vi "Lockin-4461 -Patrick -State Arrayvi.vi"(10 "IV Curve Mode":bool, 11 "Channels: AO":T6={"AO amp (V)"=[0.0, 0.0, 0.0, 0.0, 0.0, 0.0, 0.0, 0.0], "AO DC (V)"=[0.0, 0.0, 0.0, 0.0, 0.0, 0.0, 0.0, 0.0], "AO f (Hz)"=[13.0, 13.0, 13.0, 13.0, 13.0, 13.0, 13.0, 13.0], "AO phi (deg)"=[0.0, 0.0, 0.0, 0.0, 0.0, 0.0, 0.0, 0.0], "function"=[enum."Sine Wave", enum."Sine Wave", enum."Sine Wave", enum."Sine Wave", enum."Sine Wave", enum."Sine Wave", enum."Sine Wave", enum."Sine Wave"]} {"AO f (Hz)" min=0.001 max=10000.0; "AO DC (V)" format="%#_6p"; "AO amp (V)" format="%#_6p"}) -> ()   [LabVIEW 2016]
uses:
  <vilib>/Analysis/4window.llb/windowTd.ctl
  <vilib>/measure/maspectr.llb/Power Spectrum and PSD Export Mode.ctl
  <vilib>/Utility/error.llb/DialogType.ctl
  <vilib>/Analysis/baseanly.llb/Mean (DBL).vi
  <vilib>/Analysis/2dsp.llb/Decimate (single shot).vi
  <vilib>/Analysis/2dsp.llb/Decimate (single shot, DBL).vi
  <userlib>/_OpenG.lib/array/array.llb/Empty 1D Array (Variant)__ogtk.vi
  <vilib>/Platform/browser.llb/Open URL in Default Browser (string).vi
  <userlib>/_OpenG.lib/error/error.llb/Filter Error Codes (Array)__ogtk.vi
  <userlib>/_OpenG.lib/array/array.llb/Empty 1D Array (DBL)__ogtk.vi
  <vilib>/measure/maspectr.llb/FFT Power Spectrum and PSD for N Chan.vi
  <vilib>/Waveform/WDTOps.llb/WDT Waveform to XY Pairs DBL.vi
  <vilib>/measure/NI_MAPro.lvlib
  <vilib>/Analysis/NI_AALBase.lvlib
  <vilib>/Utility/config.llb/NI_LVConfig.lvlib
  <vilib>/Analysis/NI_AALPro.lvlib
panel:
  in  "Tab Control 3":enum32{"Page 1"}(tab)
  in  "Bug":bool
  in  "Trigger":bool
  in  "Notes":string
  in  "Path":path=path "C:/Data/lockin"
  in  "EXIT":bool
  in  "RESET":bool
  in  "Save Data":bool
  out "X or R":dbl=6.757945856560922e-07 caption="X or R: Current (A) or Voltage (V)" format="%#.3p"
  out "Y or Theta":dbl=134.81038545044584 caption="Y or Theta: Current (A) or Voltage (V)" format="%.3p"
  in  "Display":enum16{"X and Y", "R and Theta"}(ring)=enum."R and Theta"
  in  "Channel":dbl min=0.0 max=7.0 step=1.0
  in  "Remote Mode":bool
  out "time and date":string="22:38:56.0   2016-12-22"
  out "DAQ mode string":string="USB 4431"
  out "time since trigger":dbl
  in  "mean":dbl[](array[numeric])=[2.3266197706225262]
  in  "Tab Control 2":T1(tab)
  in  "Output signals?":bool
  out "Signals Graph":waveform(dbl)[](graph)=[{"t0"=timestamp(3565309135.890656 s since 1904-01-01), "dt"=1.0, "Y"=array[7876 elements], "attributes"=variant("NI_ChannelName"=variant(string "Dev1/ai0"), "NI_UnitDescription"=variant(string "Volts"))}]
  out "Reference Graph":waveform(dbl)[](graph)=[{"t0"=timestamp(3565309136.0036526 s since 1904-01-01), "dt"=1.0, "Y"=array[7876 elements]}, {"t0"=timestamp(3565309136.0036526 s since 1904-01-01), "dt"=1.0, "Y"=array[7876 elements]}]
  in  "decimate graph":i32=1
  in  "Display n?":bool=TRUE
  out "Display X (or R)":waveform(dbl)[](graph)=[{"t0"=timestamp(3565309135.890656 s since 1904-01-01), "dt"=1.0, "Y"=[6.757945856560922e-07]}]
  out "Display Y (or Theta)":waveform(dbl)[](graph)=[{"t0"=timestamp(3565309135.890656 s since 1904-01-01), "dt"=1.0, "Y"=[134.81038545044584]}]
  out "XY Graph":cluster{dbl[], dbl[]}[](graph)=[{[0.0, -4.762748948158435e-07], [0.0, 4.794377400353947e-07]}]
  out "Results\n(X, Y, R, Theta, mean)":dbl[][](array[numeric])=[[-4.762748948158435e-07, 4.794377400353947e-07, 6.757945856560922e-07, 134.81038545044584, 2.3266197706225262]] format="%#_3p"
  out "PS Chart":dbl[][](graph)=[[-1411.497616925462, -1404.3790029743438, -1413.0961920610762, -1418.6418791322994, -1413.136726104145, -1413.4151534226191, -1417.9246313001065, -1424.6072395567076]]
  out "PS dB":cluster{"f0":dbl, "df":dbl, "magnitude":dbl[]}[](graph)
  in  "window":T2=1 items=["Rectangle"=0, "Hanning"=1, "Hamming"=2, "Blackman-Harris"=3, "Exact Blackman"=4, "Blackman"=5, "Flat Top"=6, "4 Term B-Harris "=7, "7 Term B-Harris"=8, "Low Sidelobe"=9, "Blackman Nuttall"=11, "Triangle"=30, "Bartlett-Hanning"=31, "Bohman"=32, "Parzen"=33, "Welch"=34, "Kaiser"=60, "Dolph-Chebyshev"=61, "Gaussian"=62]
  in  "averaging parameters":T3={"averaging mode"=enum."RMS averaging", "weighting mode"=enum."Exponential", "number of averages"=10} {"number of averages" min=1}
  in  "restart averaging (F)":bool
  in  "export mode":T4 items=["Power Spectrum", "Power Spectral Density"]
  in  "window parameter":dbl=nan
  out "averages\ncompleted":dbl=8319.0
  out "averaging done":bool=TRUE
  in  "Tab Control":T5(tab)=enum."DAQ Settings"
  in  "...............reset REF":bool
  in  "............zero offset":bool
  in  "....measure offset":bool
  in  "............all  f same":bool
  in  "..........reset signal":bool
  in  "60 Hz prefilter":bool
  in  "LP prefilter":bool
  in  "LP cutoff (Hz)":dbl=30.0
  in  "Channels: Lockin":T7={"REF f (Hz)"=[13.0], "REF phi (deg)"=[0.0]} {"REF phi (deg)" format="%#_3g"}
  in  "D":dbl=0.019999999999999997 format="%.2f"
  in  "I":dbl=0.6 format="%.2f"
  in  "P":dbl=0.5 format="%.2f"
  in  "autophase?\n(experimental)":bool
  out "filter fC (Hz)":dbl=0.5305164769729844
  in  "TC (s)":dbl=0.3 format="%#_6p"
  in  "order":i32=2
  in  "save config":bool
  in  "load config":bool
  in  "Instrument":u16(ring) items=["SIMULATE", "CF900", "DR200", "MNK", "PPMS1", "PPMS2", "THz1", "THz2"]
  in  "AO Configuration":T8(array[cluster])=[{"Output physical channels"="Dev1/ao0", "AO. Max"=3.5, "AO.Min"=-3.5}]
  in  "AI Configuration":T9(array[cluster])=[{"AI.Coupling"=enum."DC", "AI.Max"=10.0, "AI.Min"=-10.0, "Input physical channels"="Dev1/ai0"}, {"AI.Coupling"=enum."DC", "AI.Max"=10.0, "AI.Min"=-10.0, "Input physical channels"="Dev1/ai1"}]
  in  "#s":i32=7876
  in  "Fs":i32=102388
  in  "auto size":bool=TRUE
  in  "decimating factor":i32=1
  in  "AI Buffer Size (S)":i32=100
  out "dt":dbl=9.766769543305856e-06 format="%#_6p"
  in  "frequency multiplier":dbl=10000.0 format="%#_13g"
  out "sampling info":cluster{"Fs":i32, "#s":i32}={"Fs"=102388, "#s"=7876}
  in  "DAQ Type":enum16{"None", "USB 4431", "PXI 446x"}(ring)=enum."USB 4431"
  in  "Amplifiers":enum16{"None", "Krohn Hite", "Femto"}(ring)
  out "Current State":string="Exit"
  out "State History":string="Macro: Initialize\rData: Initialize\rInitialize Core Data\rUI: Initialize\rUI: Front Panel State\r4461: SETUP\r4461: CREATE TASKS\rError Handler\rMacro: Exit\rData: Cleanup\rExit"
  in  "offsets":dbl[](array[numeric])=[-2.856912612915039e-05, 0.0001668522834777832, 0.00010829269886016845, 0.0027965894103050234, 0.002931471037864685, 0.0029329052329063418] format="%#.2p"
  in  "Gain":dbl[](array[numeric])=[1.0, 1.0, 1.0, 1.0, 1.0, 1.0, 1.0, 1.0]
  out "phase log":dbl[](array[numeric]) format="%.1f"
  out "AI tasks":i32
  out "AO tasks":i32
  out "error":errorcluster={"status"=TRUE, "code"=-89131, "source"="DAQmx Start Task.vi:7220017<append>\n<B>Property: </B>Start.DigEdge.Src\n<B>Property: </B>Start.DigEdge.Edge\n<B>Source Device: </B>Dev1\n<B>Source Terminal: </B>ai/StartTrigger\n\n<B>Task Name: </B>_unnamedTask<2B>"}
  # "´"
  # "Multichannel Lockin v2016/12/15 v2.0"
  # "plot 0    = AI0 f0\nplot 1    = Ai1 f0\n...\nplot N-1  = AIN f0\n\nplot N    = AI0 f1\nplot N+1  = AI1 f1\n..."
  # "AO Settings"
  # "Lockin Settings"
  # "prefilters"
  # "lockin filter"
  # "autophase"
  # "0"
  # "1"
  # "2"
  # "3"
  # "4"
  # "5"
  # "6"
  # "7"
  # "configuration"
  # "sampling"
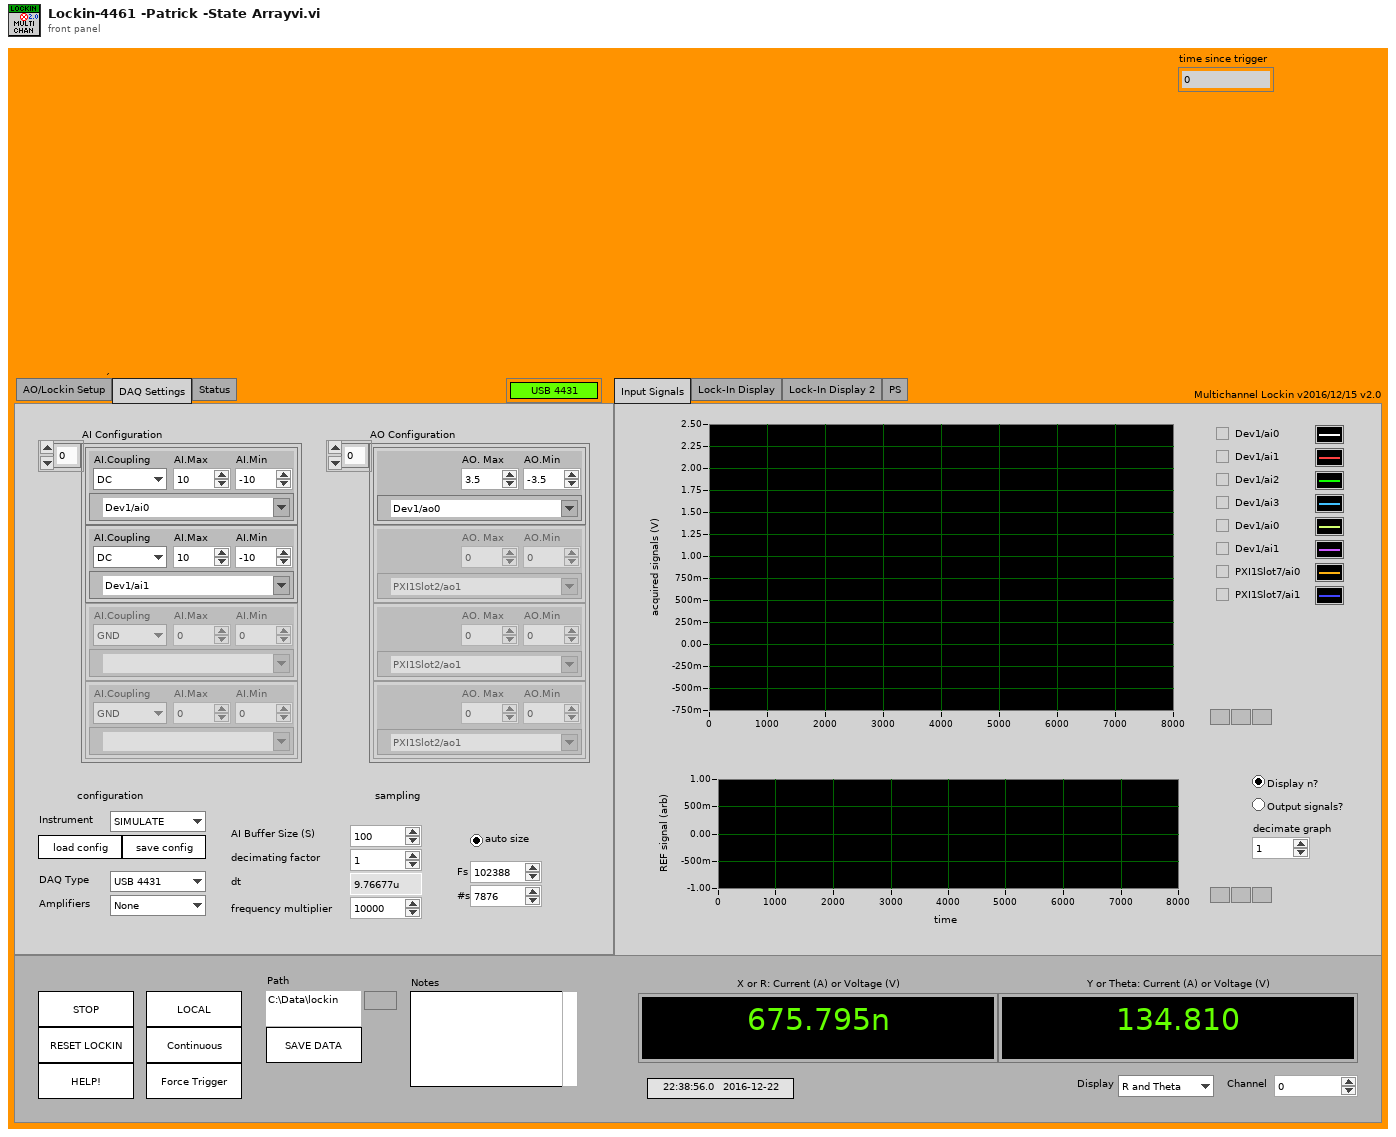
[diagram p1: front panel]
types:
  T1 = enum32{"Input Signals", "Lock-In Display", "Lock-In Display 2", "PS"}
  T2 = typedef "NI_AALPro.lvlib/windowTd.ctl" = u32
  T3 = cluster{"averaging mode":enum16{"No averaging", "Vector averaging", "RMS averaging", "Peak hold"}, "weighting mode":enum16{"Linear", "Exponential"}, "number of averages":u32}
  T4 = typedef "NI_MAPro.lvlib/Power Spectrum and PSD Export Mode.ctl" = u16
  T5 = enum32{"AO/Lockin Setup", "DAQ Settings", "Status"}
  T6 = cluster{"AO amp (V)":dbl[], "AO DC (V)":dbl[], "AO f (Hz)":dbl[], "AO phi (deg)":dbl[], "function":enum16{"Sine Wave", "Triangle Wave", "Square Wave", "Sawtooth Wave"}[]}
  T7 = cluster{"REF f (Hz)":dbl[], "REF phi (deg)":dbl[]}
  T8 = cluster{"Output physical channels":tag, "AO. Max":dbl, "AO.Min":dbl}[]
  T9 = cluster{"AI.Coupling":enum16{"AC", "DC", "GND"}, "AI.Max":dbl, "AI.Min":dbl, "Input physical channels":tag}[]
  T10 = enum32{"invalid app kind", "Development System", "Run Time System", "Student Edition", "Embedded LabVIEW", "Evaluation", "Custom"}
  T11 = enum32{"Invalid", "Standard", "Closed", "Hidden", "Minimized", "Maximized"}
  T12 = enum32{"Input Signals", "Lock-In Display", "Lock-In Display 2", "PS", "FFT"}
  T13 = cluster{"Core":cluster{"Current VI Reference":refnum<vi>, "Close Panel on Exit?":bool}, "Error":bool, "Your string data":string, "AI task":refnum<k21>[], "AO task":refnum<k21>[], "Input Signals":waveform(dbl)[], "Ouput Signals":waveform(dbl)[], "REF":waveform(dbl)[], "sampling info":cluster{"Fs":dbl, "#s":dbl}, "Tasks":string[]}
  T14 = typedef "DialogType.ctl" = u16
  T15 = cluster{"Current VI Reference":refnum<vi>, "Close Panel on Exit?":bool}
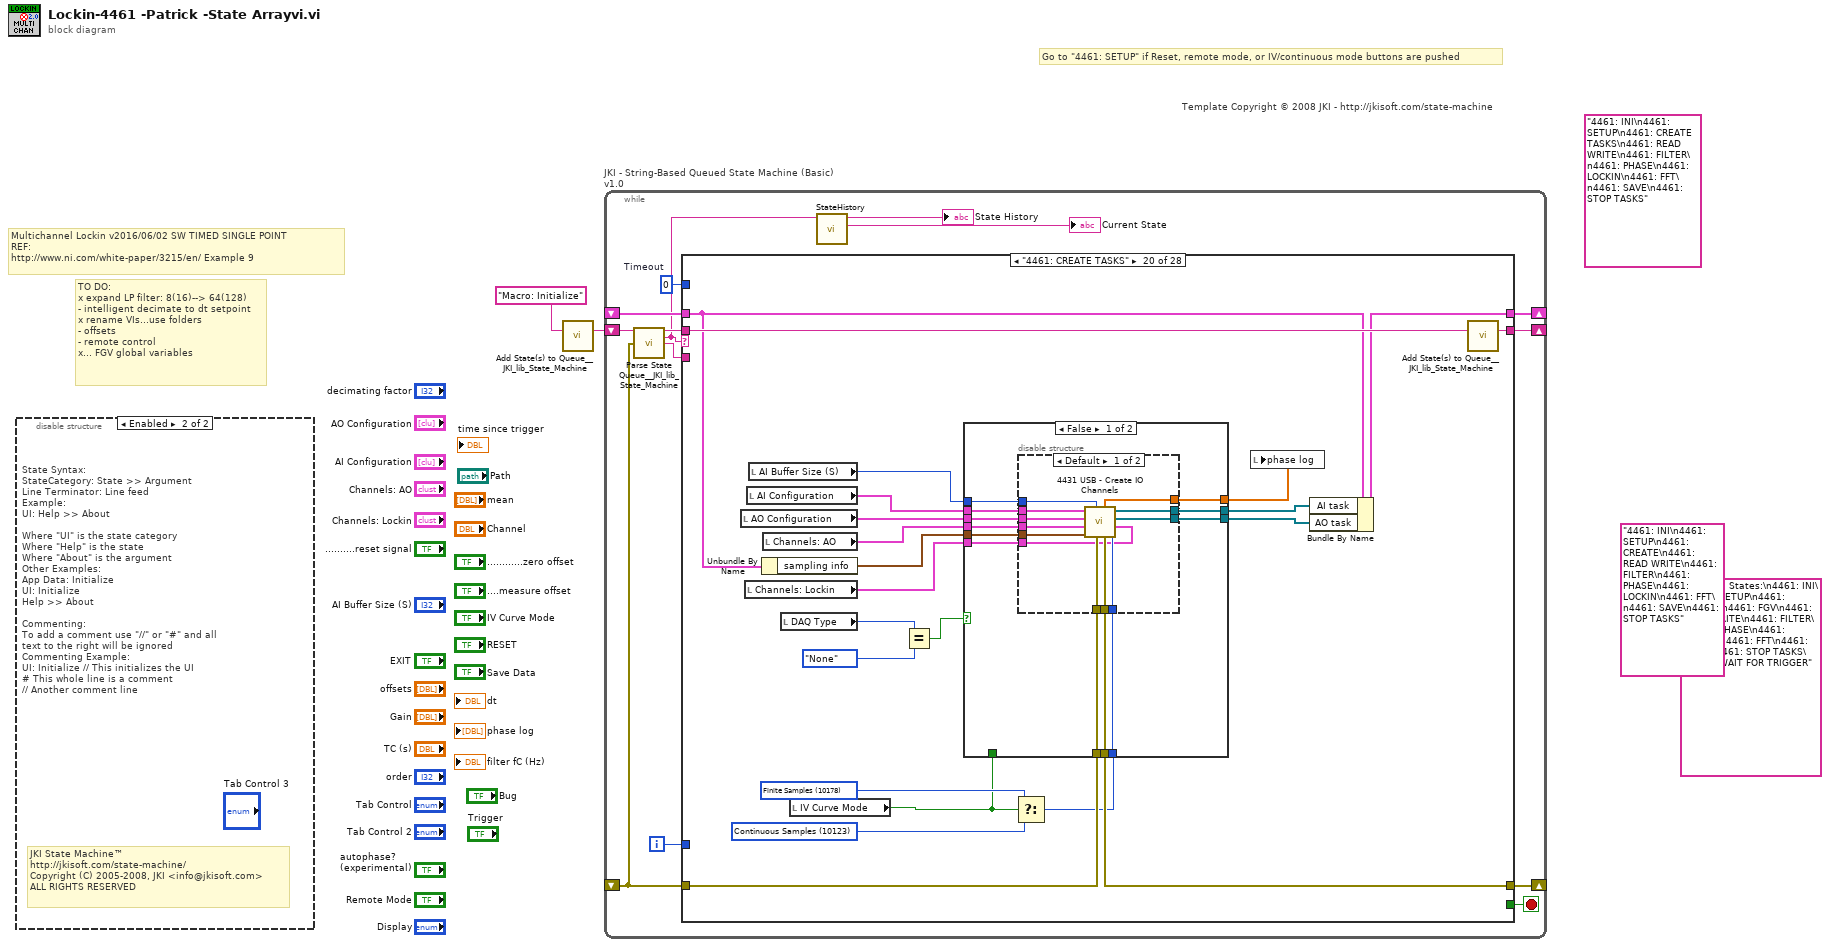
[diagram p0: block diagram]
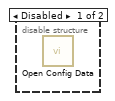
[diagram p2: hidden frame]
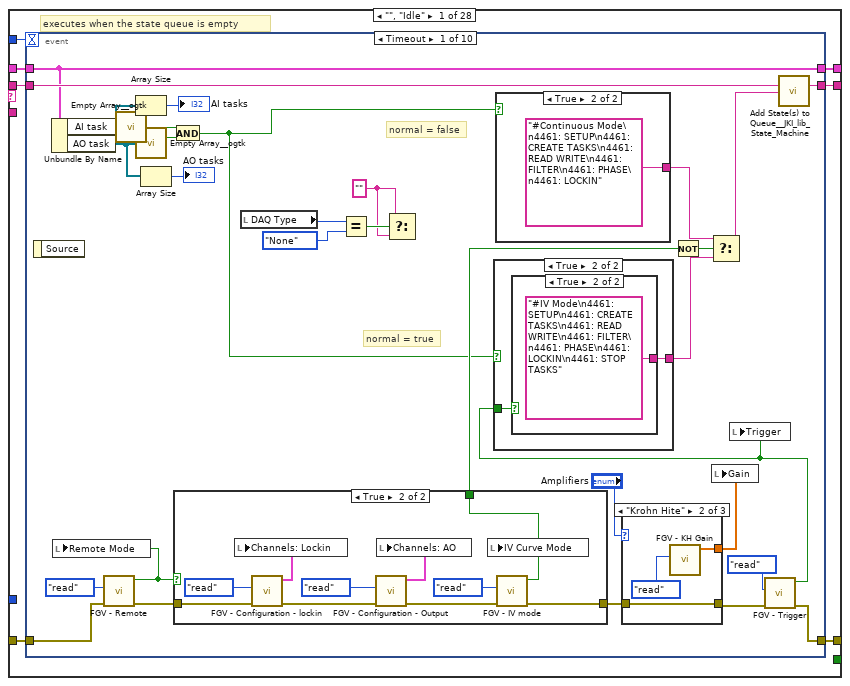
[diagram p3: hidden frame]
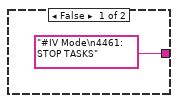
[diagram p4: hidden frame]
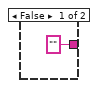
[diagram p5: hidden frame]
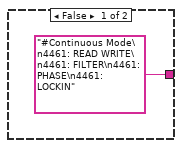
[diagram p6: hidden frame]
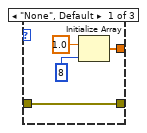
[diagram p7: hidden frame]
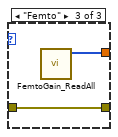
[diagram p8: hidden frame]
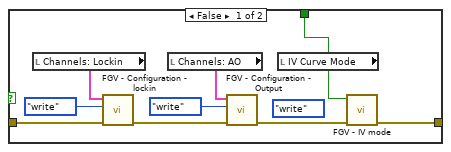
[diagram p9: hidden frame]
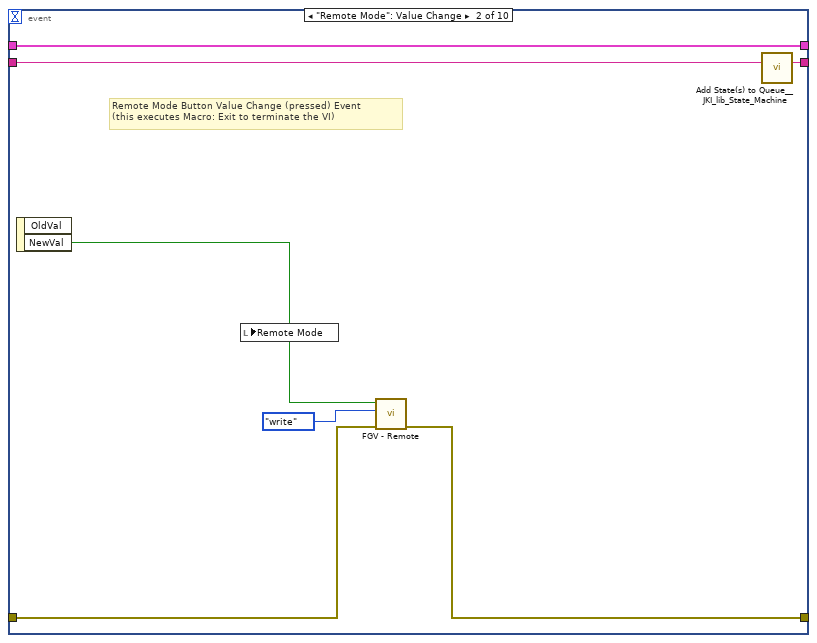
[diagram p10: hidden frame]
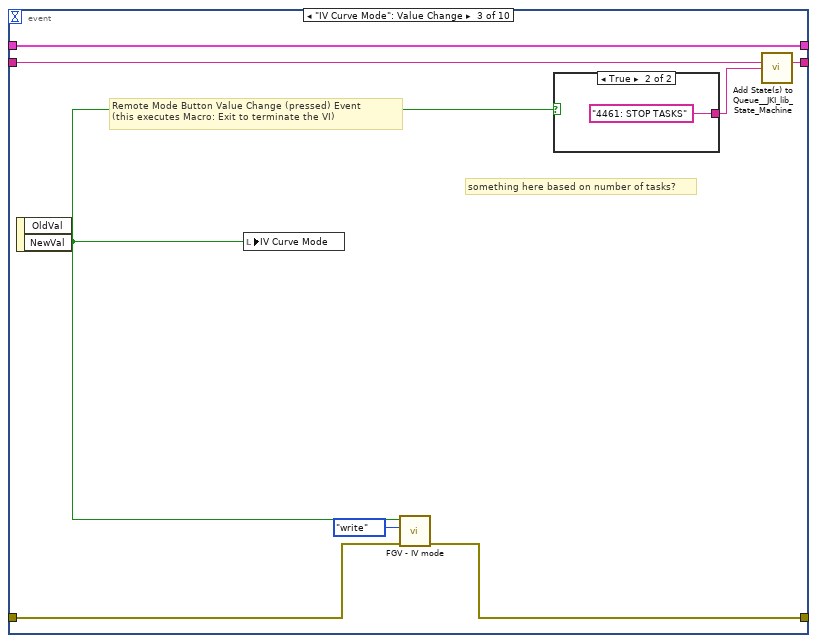
[diagram p11: hidden frame]
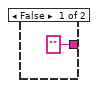
[diagram p12: hidden frame]
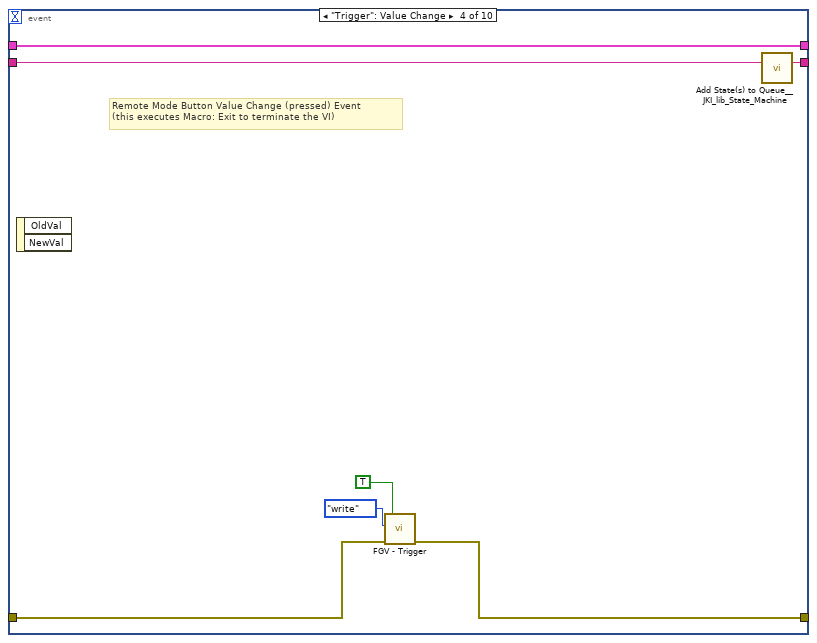
[diagram p13: hidden frame]
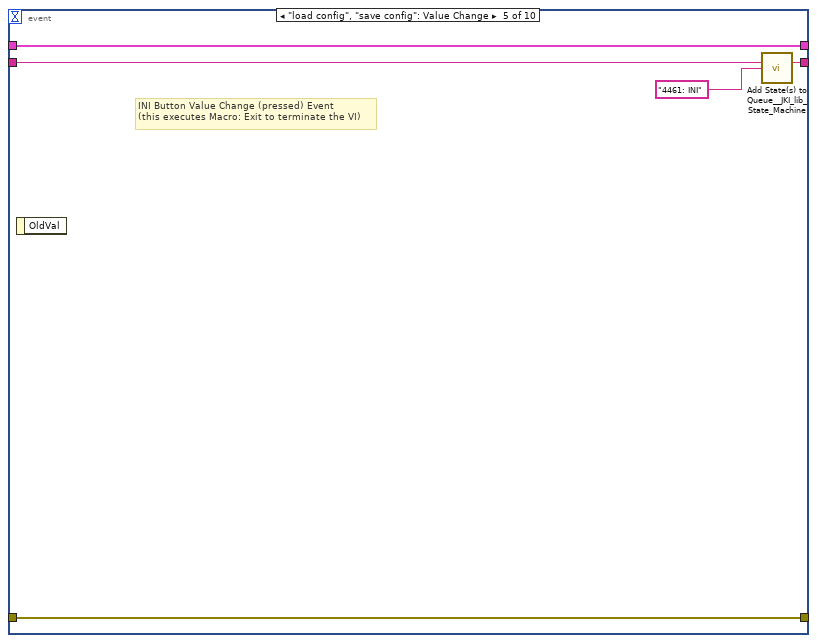
[diagram p14: hidden frame]
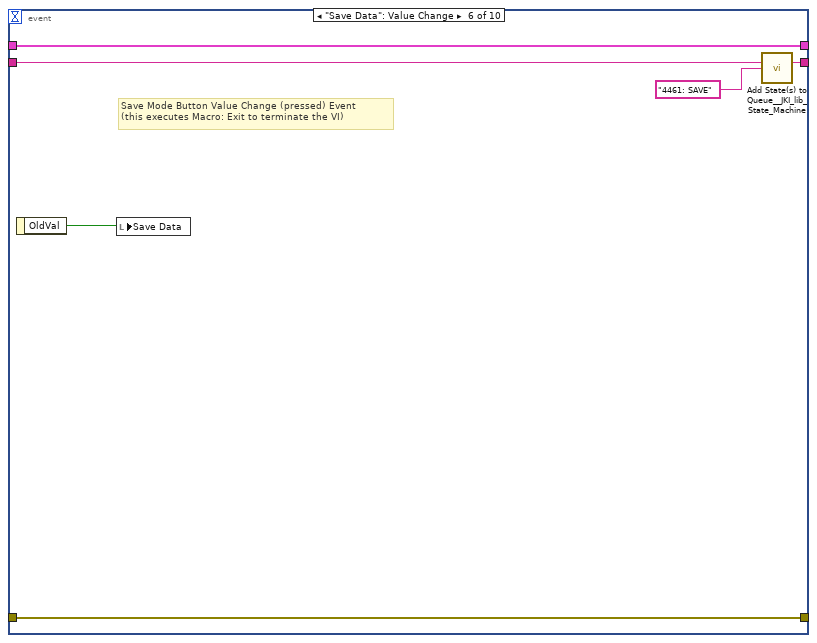
[diagram p15: hidden frame]
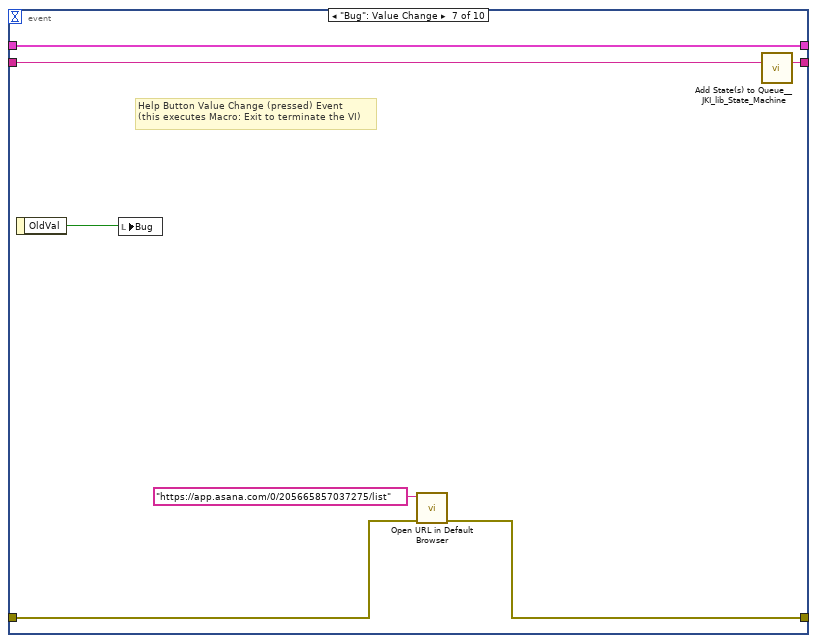
[diagram p16: hidden frame]
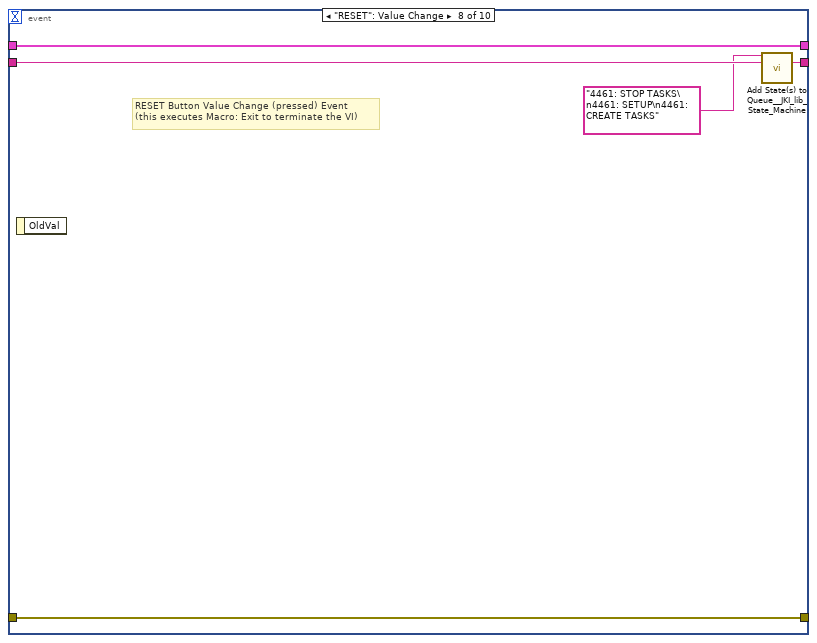
[diagram p17: hidden frame]
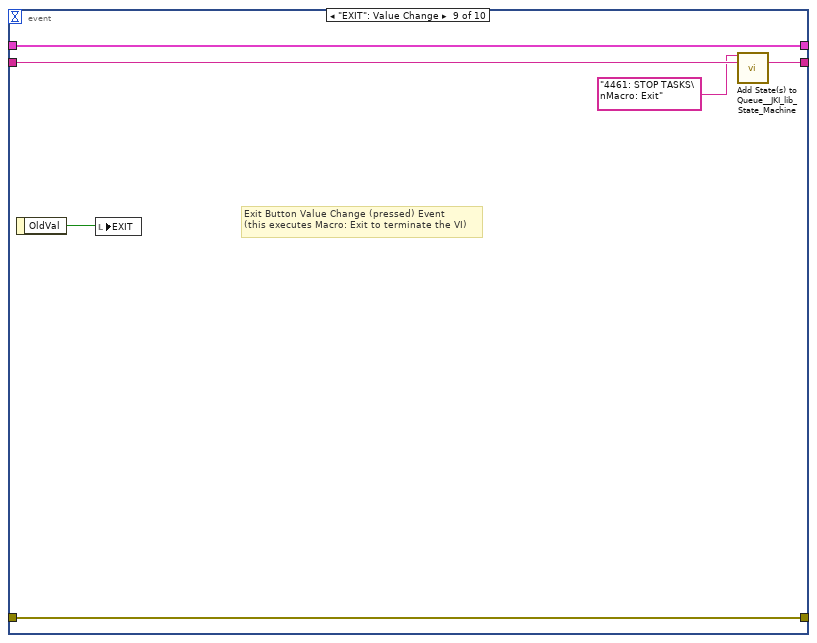
[diagram p18: hidden frame]
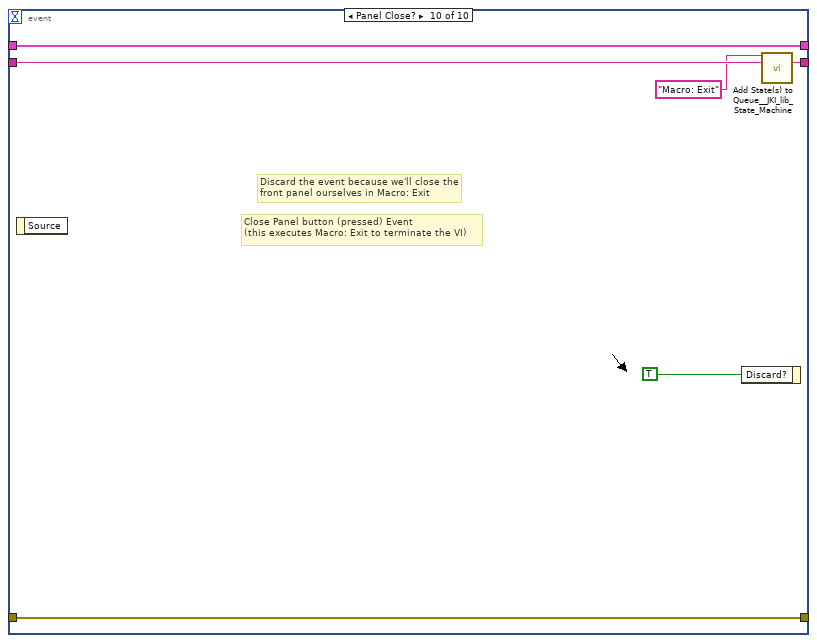
[diagram p19: hidden frame]
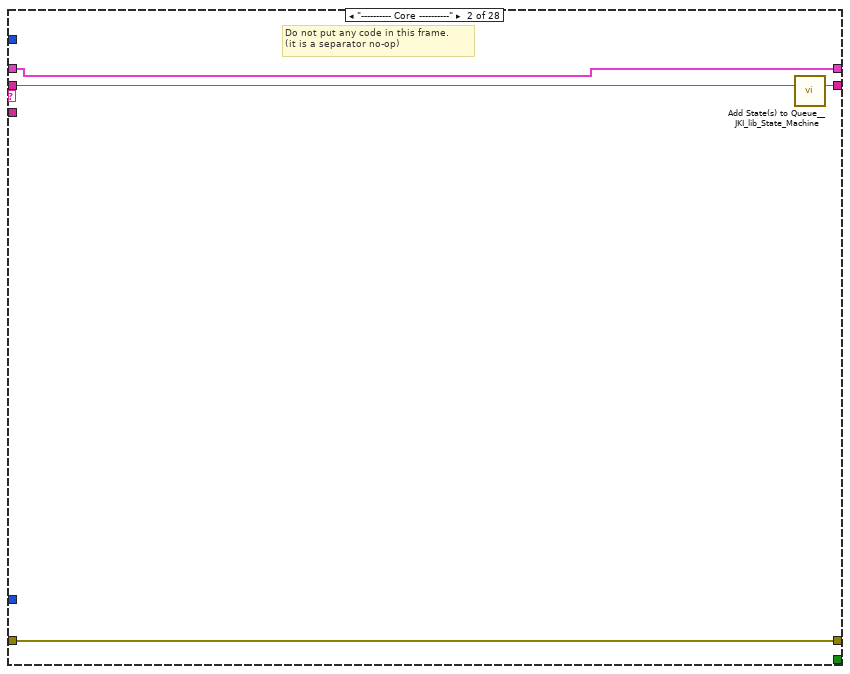
[diagram p20: hidden frame]
diagram:
  (unwired) "4461: INI\n4461: SETUP\n4461: CREATE\n4461: READ WRITE\n4461: FILTER\n4461: PHASE\n4461: LOCKIN\n4461: FFT\n4461: SAVE\n4461: STOP TASKS" ("State(s) at Back (\"\")")
  (unwired) "All 4461 States:\n4461: INI\n4461: SETUP\n4461: CREATE\n4461: FGV\n4461: READ WRITE\n4461: FILTER\n4461: PHASE\n4461: LOCKIN\n4461: FFT\n4461: SAVE\n4461: STOP TASKS\n4461: WAIT FOR TRIGGER" ("State(s) at Back (\"\")")
  (unwired) "4461: INI\n4461: SETUP\n4461: CREATE TASKS\n4461: READ WRITE\n4461: FILTER\n4461: PHASE\n4461: LOCKIN\n4461: FFT\n4461: SAVE\n4461: STOP TASKS" ("State(s) at Back (\"\")")
  # "Template Copyright © 2008 JKI - http://jkisoft.com/state-machine"
  # "Go to \"4461: SETUP\" if Reset, remote mode, or IV/continuous mode buttons are pushed"
  # "Multichannel Lockin v2016/06/02 SW TIMED SINGLE POINT\nREF:\nhttp://www.ni.com/white-paper/3215/en/ Example 9"
  # "TO DO:\nx expand LP filter: 8(16)--> 64(128)\n- intelligent decimate to dt setpoint\nx rename VIs...use folders\n- offsets\n- remote control\nx... FGV global variables"
  n1 = disable-structure shown="Enabled" {
    frame Disabled {
      n2 = call <vilib>:"Open Config Data.vi"() -> ()  [unwired: 9 in, 3 out]
    }
    frame Enabled {
      # "JKI State Machine™\nhttp://jkisoft.com/state-machine/\nCopyright (C) 2005-2008, JKI <info@jkisoft.com>\nALL RIGHTS RESERVED"
      # "State Syntax:\nStateCategory: State >> Argument\nLine Terminator: Line feed\nExample:\nUI: Help >> About\n\nWhere \"UI\" is the state category\nWhere \"Help\" is the state\nWhere \"About\" is the argument\nOther Examples:\nApp Data: Initialize\nUI: Initialize\nHelp >> About\n\nCommenting:\nTo add a comment use \"//\" or \"#\" and all text to the right will be ignored\nCommenting Example:\nUI: Initialize // This initializes the UI\n# This whole line is a comment\n// Another comment line"
    }
  }
  n3 = call <vilib>:"Add State(s) to Queue__JKI_lib_State_Machine.vi"("State(s) in (\"\")"="Macro: Initialize") -> ("States Out"=w2:string)  [unwired: 14 in]
  n4 = while "JKI - String-Based Queued State Machine (Basic) v1.0" {
    shift-right: [w5] -> _
    shift-left: _ -> [w6]
    shift-right: [w15] -> _
    shift-left: _ -> [w7]
    shift-right: [w14] -> _
    shift-left: w2 -> [w8]
    i -> [w10]
    stop <- w13 stop-if-true
    w12 = 0  # Timeout
    n5 = call <vilib>:"Parse State Queue__JKI_lib_State_Machine.vi"("State Queue"=w8, "Error In (no error)"=w7) -> ("Remaining States"=w11:string, "Current State"=w3:string, "Arguments"=w16:string)  [unwired: 11 in]
    n6 = case shown="\"4461: CREATE TASKS\"" w3 {
      selector: w3 -> [_ _ w152 _ _ _ _ _ _ _ _ _ _ _ _ _ _ _ _ _ _ _ _ _ _ _ _ _]
      tunnel: w16 -> [_ _ _ _ _ _ _ _ _ _ _ w231 w242 _ _ _ _ _ _ _ _ _ _ _ _ _ _ _]
      tunnel: w6 -> [w21 w148 w154 w165 w180 w192 w195 _ w213 w219 w226 w230 w241 w269 w273 w278 w289 w298 w339 w378 w459 w508 w563 w626 w649 w697 w725 w774]
      tunnel: [w20 w149 w158 w171 errorcluster {"status"=FALSE, "code"=0, "source"=""} ("error out") w191 w196 w209 w214 w220 w224 w232 w240 w270 w275 w286 w290 w295 w328 w380 w467 w519 w552 w627 w651 w687 w726 w773] -> w15
      tunnel: w7 -> [w19 w149 w157 w171 w177 w191 w196 w209 w215 w220 w224 w233 w244 w270 w275 w286 w290 w296 w328 w384 w469 w522 w552 w627 w651 w686 w736 w773]
      tunnel: [w22 w150 w155 w173 w184 w193 w197 w211 w217 w221 w228 w234 w245 w271 w276 w287 w291 w300 w342 w390 w471 w530 w564 w625 w650 w698 w722 w771] -> w14
      tunnel: [_ _ _ _ _ TRUE _ _ _ _ _ _ _ _ _ _ _ _ _ _ _ _ _ _ _ _ _ _] -> w13
      tunnel: [w18 w148 w154 w172 w181 w192 w195 w210 w213 w219 w226 w230 w241 w269 w273 w278 w289 w298 w337 w385 w470 w529 w563 w626 w649 w697 w724 w774] -> w5
      tunnel: w12 -> [w17 _ _ _ _ _ _ _ _ _ _ _ _ _ _ _ _ _ _ _ _ _ _ _ _ _ _ _]
      tunnel: w11 -> [w23 w151 w156 w174 w185 w194 w198 w212 w218 w222 w229 w235 w246 w272 w277 w288 w292 w299 w343 w391 w472 w531 w565 w628 w652 w699 w737 w775]
      tunnel: w10 -> [_ _ _ _ _ _ _ _ _ _ _ _ _ _ _ _ _ _ _ _ _ _ _ _ _ _ _ _]
      frame "", "Idle" {
        # "executes when the state queue is empty"
        n7 = event shown="[0] Timeout" {
          selector: _ -> [_ _ _ _ _ _ _ _ _ _]
          dyn-events: _ -> [_ _ _ _ _ _ _ _ _ _]
          timeout: w17 -> [_ _ _ _ _ _ _ _ _ _]
          tunnel: w23 -> [w53 w95 w103 w112 w117 w123 w130 w135 w141 w147]
          tunnel: [w52 w94 w102 w111 w116 w122 w129 w134 w140 w146] -> w22
          tunnel: w21 -> [w40 w93 w101 w110 w115 w121 w128 w133 w138 w144]
          tunnel: [w41 w90 w98 w106 w113 w120 w125 w132 w139 w145] -> w20
          tunnel: w19 -> [w50 w91 w99 w107 w113 w120 w127 w132 w139 w145]
          tunnel: [w40 w93 w101 w110 w115 w121 w128 w133 w138 w144] -> w18
          event Timeout {
            w26 = "" ("State(s) at Back (\"\")")
            # "normal = true"
            # "normal = false"
            n8 = event-data() -> ()  [unwired: 1 in, 1 out]
            n9 = Unbundle By Name(w40) -> ("AI task"=w32:refnum<k21>[], "AO task"=w30:refnum<k21>[])
            n10 = call "FGV - Remote.vi"("error in"=w50, "Function"=enum16{"write", "read"}."read") -> ("error out"=w48:errorcluster, "Remote Mode"=w43:bool)  [unwired: 4 in]
            n11 = local write "Remote Mode"(w43) -> ()
            n12 = call-poly <userlib>:"Empty Array__ogtk.vi"("Array"=w32) -> ("Empty Array?"=w39:bool)  [unwired: 8 in]
            n13 = Array Size(array=w32) -> (size(s)=→"AI tasks":i32)
            n14 = call-poly <userlib>:"Empty Array__ogtk.vi"("Array"=w30) -> ("Empty Array?"=w38:bool)  [unwired: 8 in]
            n15 = Array Size(array=w30) -> (size(s)=→"AO tasks":i32)
            n16 = And(x=w39, y=w38) -> (x .and. y?=w27:bool)
            n17 = case shown="True" w43 {
              tunnel: [w72 w82] -> w47
              tunnel: w48 -> [w74 w85]
              tunnel: [w70 w79] -> w46
              frame False {
                (unwired) enum16{"write", "read"}."write" ("Function")
                n18 = local read "Channels: Lockin"() -> (w75:T7)
                n19 = call "FGV - Configuration - lockin.vi"("error in"=w74, "Function"=enum16{"write", "read"}."write", "Channels: Lockin"=w75) -> ("error out"=w76:errorcluster)  [unwired: 3 in, 1 out]
                n20 = local read "Channels: AO"() -> (w71:T6)
                n21 = call "FGV - Configuration - Output.vi"("error in"=w76, "Function"=enum16{"write", "read"}."write", "Channels: AO"=w71) -> ("error out"=w73:errorcluster)  [unwired: 3 in, 1 out]
                n22 = local read "IV Curve Mode"() -> (w70:bool)
                n23 = call "FGV - IV mode.vi"("error in"=w73, "IV mode"=w70) -> ("error out"=w72:errorcluster)  [unwired: 4 in, 1 out]
              }
              frame True {
                n24 = call "FGV - Configuration - lockin.vi"("error in"=w85, "Function"=enum16{"write", "read"}."read") -> ("error out"=w86:errorcluster, "Channels: Lockin 2"=w84:T7)  [unwired: 4 in]
                n25 = local write "Channels: Lockin"(w84) -> ()
                n26 = call "FGV - Configuration - Output.vi"("error in"=w86, "Function"=enum16{"write", "read"}."read") -> ("error out"=w83:errorcluster, "Channels: AO 2"=w81:T6)  [unwired: 4 in]
                n27 = local write "Channels: AO"(w81) -> ()
                n28 = call "FGV - IV mode.vi"("error in"=w83, "Function"=enum16{"write", "read"}."read") -> ("error out"=w82:errorcluster, "IV mode"=w79:bool)  [unwired: 4 in]
                n29 = local write "IV Curve Mode"(w79) -> ()
              }
            }
            n30 = local read "DAQ Type"() -> (w35:enum16{"None", "USB 4431", "PXI 446x"})
            n31 = Equal?(x=w35, y=enum16{"None", "USB 4431", "PXI 446x"}."None" ("DAQ Type")) -> (x = y?=w33:bool)
            n32 = Select(t=w26, s=w33, f=w26) -> ()  [unwired: 1 out]
            n33 = case shown="True" w27 {
              tunnel: ["#Continuous Mode\n4461: READ WRITE\n4461: FILTER\n4461: PHASE\n4461: LOCKIN" ("State(s) at Back (\"\")") "#Continuous Mode\n4461: SETUP\n4461: CREATE TASKS\n4461: READ WRITE\n4461: FILTER\n4461: PHASE\n4461: LOCKIN" ("State(s) at Back (\"\")")] -> w28
              frame False {
              }
              frame True {
              }
            }
            n34 = case shown="\"Krohn Hite\"" "Amplifiers" {
              tunnel: [w62 w67 w68] -> w42
              tunnel: [w63 w66 w69] -> w49
              tunnel: w47 -> [w62 w67 w68]
              frame "None", Default {
                n35 = Initialize Array(1.0 ("element"), 8 ("dimension size")) -> (w63:dbl[])
              }
              frame "Krohn Hite" {
                n36 = call <userlib>:"FGV - KH Gain.vi"("Function"=enum16{"write", "read"}."read") -> ("Array 2"=w66:dbl[])  [unwired: 5 in, 1 out]
              }
              frame "Femto" {
                n37 = call <userlib>:"FemtoGain_ReadAll.vi"() -> ("Femto Gains"=w69:i32[])  [unwired: 11 in]
              }
            }
            n38 = Not(x=w46) -> (.not. x?=w36:bool)
            n39 = local write "Gain"(w49) -> ()
            n40 = call "FGV - Trigger.vi"("error in"=w42, "Function"=enum16{"write", "read"}."read") -> ("error out"=w41:errorcluster, "Trigger 2"=w24:bool)  [unwired: 4 in]
            n41 = case shown="True" w27 {
              tunnel: ["#IV Mode\n4461: STOP TASKS" ("State(s) at Back (\"\")") w56] -> w44
              tunnel: w24 -> [_ w55]
              frame False {
              }
              frame True {
                n42 = case shown="True" w55 {
                  tunnel: ["" ("State(s) at Back (\"\")") "#IV Mode\n4461: SETUP\n4461: CREATE TASKS\n4461: READ WRITE\n4461: FILTER\n4461: PHASE\n4461: LOCKIN\n4461: STOP TASKS" ("State(s) at Back (\"\")")] -> w56
                  frame False {
                  }
                  frame True {
                  }
                }
              }
            }
            n43 = Select(t=w28, s=w36, f=w44) -> (s? t:f=w37:string)
            n44 = local write "Trigger"(w24) -> ()
            n45 = call <vilib>:"Add State(s) to Queue__JKI_lib_State_Machine.vi"("State(s) in (\"\")"=w53, "State(s) at Back (\"\")"=w37) -> ("States Out"=w52:string)  [unwired: 13 in]
          }
          event "Remote Mode": Value Change {
            # "Remote Mode Button Value Change (pressed) Event\n(this executes Macro: Exit to terminate the VI)"
            n46 = event-data() -> ("NewVal"=w89:bool)  [unwired: 1 in, 1 out]
            n47 = local write "Remote Mode"(w89) -> ()
            n48 = call "FGV - Remote.vi"("error in"=w91, "Function"=enum16{"write", "read"}."write", "Remote Mode"=w89) -> ("error out"=w90:errorcluster)  [unwired: 3 in, 1 out]
            n49 = call <vilib>:"Add State(s) to Queue__JKI_lib_State_Machine.vi"("State(s) in (\"\")"=w95) -> ("States Out"=w94:string)  [unwired: 14 in]
          }
          event "IV Curve Mode": Value Change {
            # "something here based on number of tasks?"
            # "Remote Mode Button Value Change (pressed) Event\n(this executes Macro: Exit to terminate the VI)"
            n50 = event-data() -> ("NewVal"=w96:bool)  [unwired: 1 in, 1 out]
            n51 = local write "IV Curve Mode"(w96) -> ()
            n52 = call "FGV - IV mode.vi"("error in"=w99, "Function"=enum16{"write", "read"}."write", "IV mode"=w96) -> ("error out"=w98:errorcluster)  [unwired: 3 in, 1 out]
            n53 = case shown="True" w96 {
              tunnel: ["" ("State(s) at Back (\"\")") "4461: STOP TASKS" ("State(s) at Back (\"\")")] -> w97
              frame False {
              }
              frame True {
              }
            }
            n54 = call <vilib>:"Add State(s) to Queue__JKI_lib_State_Machine.vi"("State(s) in (\"\")"=w103, "State(s) at Back (\"\")"=w97) -> ("States Out"=w102:string)  [unwired: 13 in]
          }
          event "Trigger": Value Change {
            # "Remote Mode Button Value Change (pressed) Event\n(this executes Macro: Exit to terminate the VI)"
            n55 = event-data() -> ()  [unwired: 1 in, 2 out]
            n56 = call "FGV - Trigger.vi"("error in"=w107, "Function"=enum16{"write", "read"}."write", "Trigger"=TRUE) -> ("error out"=w106:errorcluster)  [unwired: 3 in, 1 out]
            n57 = call <vilib>:"Add State(s) to Queue__JKI_lib_State_Machine.vi"("State(s) in (\"\")"=w112) -> ("States Out"=w111:string)  [unwired: 14 in]
          }
          event "load config", "save config": Value Change {
            # "INI Button Value Change (pressed) Event\n(this executes Macro: Exit to terminate the VI)"
            n58 = event-data() -> ()  [unwired: 1 in, 1 out]
            n59 = call <vilib>:"Add State(s) to Queue__JKI_lib_State_Machine.vi"("State(s) in (\"\")"=w117, "State(s) at Back (\"\")"="4461: INI") -> ("States Out"=w116:string)  [unwired: 13 in]
          }
          event "Save Data": Value Change {
            # "Save Mode Button Value Change (pressed) Event\n(this executes Macro: Exit to terminate the VI)"
            n60 = event-data() -> ("OldVal"=w118:bool)  [unwired: 1 in]
            n61 = local write "Save Data"(w118) -> ()
            n62 = call <vilib>:"Add State(s) to Queue__JKI_lib_State_Machine.vi"("State(s) in (\"\")"=w123, "State(s) at Back (\"\")"="4461: SAVE") -> ("States Out"=w122:string)  [unwired: 13 in]
          }
          event "Bug": Value Change {
            # "Help Button Value Change (pressed) Event\n(this executes Macro: Exit to terminate the VI)"
            n63 = event-data() -> ("OldVal"=w124:bool)  [unwired: 1 in]
            n64 = local write "Bug"(w124) -> ()
            n65 = call-poly <vilib>:"Open URL in Default Browser.vi"("error in (no error)"=w127, "URL"="https://app.asana.com/0/205665857037275/list") -> ("error out"=w125:errorcluster)  [unwired: 4 in, 1 out]
            n66 = call <vilib>:"Add State(s) to Queue__JKI_lib_State_Machine.vi"("State(s) in (\"\")"=w130) -> ("States Out"=w129:string)  [unwired: 14 in]
          }
          event "RESET": Value Change {
            # "RESET Button Value Change (pressed) Event\n(this executes Macro: Exit to terminate the VI)"
            n67 = event-data() -> ()  [unwired: 1 in, 1 out]
            n68 = call <vilib>:"Add State(s) to Queue__JKI_lib_State_Machine.vi"("State(s) in Front (\"\")"="4461: STOP TASKS\n4461: SETUP\n4461: CREATE TASKS", "State(s) in (\"\")"=w135) -> ("States Out"=w134:string)  [unwired: 13 in]
          }
          event "EXIT": Value Change {
            # "Exit Button Value Change (pressed) Event\n(this executes Macro: Exit to terminate the VI)"
            n69 = event-data() -> ("OldVal"=w136:bool)  [unwired: 1 in]
            n70 = local write "EXIT"(w136) -> ()
            n71 = call <vilib>:"Add State(s) to Queue__JKI_lib_State_Machine.vi"("State(s) in Front (\"\")"="4461: STOP TASKS\nMacro: Exit", "State(s) in (\"\")"=w141) -> ("States Out"=w140:string)  [unwired: 13 in]
          }
          event Panel Close? {
            # "Discard the event because we'll close the front panel ourselves in Macro: Exit"
            # "Close Panel button (pressed) Event\n(this executes Macro: Exit to terminate the VI)"
            n72 = event-data() -> ()  [unwired: 1 in, 1 out]
            n73 = event-data("Discard?"=TRUE) -> ()  [unwired: 1 in, 1 out]
            n74 = call <vilib>:"Add State(s) to Queue__JKI_lib_State_Machine.vi"("State(s) in Front (\"\")"="Macro: Exit", "State(s) in (\"\")"=w147) -> ("States Out"=w146:string)  [unwired: 13 in]
          }
        }
      }
      frame "---------- Core ----------" {
        # "Do not put any code in this frame.\n(it is a separator no-op)"
        n75 = call <vilib>:"Add State(s) to Queue__JKI_lib_State_Machine.vi"("State(s) in (\"\")"=w151) -> ("States Out"=w150:string)  [unwired: 14 in]
      }
      frame Default {
        w161 = 42 items=["No error", "Argument error", "Memory is full", "Out of zone", "End of file", "File already open", "Generic file I/O error", "File not found", "File permission error", "Disk is full", "Duplicate path", "Too many files open", "System feature not enabled", "Resource file not found", "Cannot add resource", "Resource not found", "Image not found", "Image memory error", "Pen does not exist", "Config type invalid", "Config token not found", "Config parse error", "Config memory error", "Bad external code format", "Bad external code offset", "External code not present", "Null window", "Destroy window error", "Null menu", "Print aborted", "Bad print record", "Print driver error", "Windows error during printing", "Memory error during printing", "Print dialog error", "Generic print error", "Invalid device refnum", "Device not found", "Device parameter error", "Device unit error", "Cannot open device", "Device call aborted", "Generic error", "Cancelled by user", "Object ID too low", "Object ID too high", "Object not in heap", "Unknown heap", "Unknown object (invalid DefProc)", "Unknown object (DefProc not in table)", "Message out of range", "Invalid (null) method", "Unknown message", "Manager call not supported", "Bad address", "Network operation in progress", "Network operation timed out", "Connection is busy", "Network attribute not supported", "Network error", "Address in use", "System out of memory", "Connection aborted", "Connection refused", "Not connected", "Already connected", "Connection closed", "Initialization error (interapplication manager)", "Bad occurrence", "Wait on unbound occurrence handler", "Occurrence queue overflow", "Datalog type conflict", "Unused", "Unrecognized type (interapplication manager)", "Memory corrupt", "Failed to make temporary DLL", "Old CIN version", "Drag socket not found", "Failed to load drop-object", "Failed to register OLE object", "Failed to release OLE object", "Format specifier type mismatch", "Unknown format specifier", "Too few format specifiers", "Too many format specifiers", "Scan failed", "Newer CIN version", "Error converting to variant", "Runtime menu error", "Password tampered", "Variant attribute not found", "Incompatible variant data type", "Event data is not available", "Event Store is not present", "Occurrence is not found", "Event Queue is not created", "Event info is not available", "Refnum passed is NULL", "Error retrieving Class GUID", "Error retrieving CoClass GUID", "Error retrieving TypeLib GUID.", "Bad built application magic bytes.", "Specific driver is different from the specific driver associated with the Logical Name.", "There is no session opened to the class driver.", "Max Error", "MAX - Error with config objects", "MAX - Error loading configuration", "MAX - Group not supported"]
        # "Current State"
        # "Do not delete, rename, or modify this frame.\n(this is used to capture unhandled states and typos)"
        # "Handle mistyped state name (developer tool)"
        n76 = Format Into String(format string="Software Exception: Unhandled State \"%s\"." ("message"), error in=w157, w152) -> (resulting string=w160:string, error out=w159:errorcluster)  [unwired: 1 in]
        n77 = call <vilib>:"Error Cluster From Error Code.vi"("show call chain? (False)"=TRUE, "error in (no error)"=w159, "error message (\"\")"=w160, "error code (0)"=w161) -> ("error out"=w158:errorcluster)  [unwired: 5 in]
        n78 = call <vilib>:"Add State(s) to Queue__JKI_lib_State_Machine.vi"("State(s) in (\"\")"=w156) -> ("States Out"=w155:string)  [unwired: 14 in]
      }
      frame "Initialize Core Data" {
        # "Do not delete, rename, or modify this frame.\n(this is used to determine panel behavior on exit)"
        # "originally closed?"
        # "exe?"
        # "If panel starts closed or is an EXE, then close it when we exit"
        n79 = property class="VI"() -> ("Front Panel.Open"=w170:bool)  [unwired: 2 in, 2 out]
        n80 = property class="App"() -> ("App.Kind"=w169:T10)  [unwired: 2 in, 2 out]
        n81 = control-ref of="Current VI Reference"() -> (w163:refnum<vi>)
        n82 = Not(x=w170) -> (.not. x?=w167:bool)
        n83 = Equal?(x=w169, y=T10."Run Time System" ("Application:Kind")) -> (x = y?=w166:bool)
        n84 = Or(x=w167, y=w166) -> (x .or. y?=w164:bool)
        n85 = Bundle By Name(cluster=w165, "Core.Current VI Reference"=w163, "Core.Close Panel on Exit?"=w164) -> (w172:T13)
        n86 = call <vilib>:"Add State(s) to Queue__JKI_lib_State_Machine.vi"("State(s) in (\"\")"=w174) -> ("States Out"=w173:string)  [unwired: 14 in]
      }
      frame "Error Handler" {
        # "Handle any errors here.\nYou can also output any states to clean-up after errors occur"
        # "Clear error"
        n87 = Unbundle By Name(w180) -> ("Error"=w182:bool)
        n88 = Not(x=w182) -> (.not. x?=w175:bool)
        n89 = Bundle By Name(cluster=w180, "Error"=w175) -> (w181:T13)
        n90 = call-poly <userlib>:"Filter Error Codes__ogtk.vi"("Error In"=w177, "Error Codes to Filter"=i32[] [-200077]) -> ("Error Out"=w176:errorcluster)  [unwired: 7 in, 2 out]
        n91 = case shown="No Error" w176 {
          selector: w176 -> [_ w188]
          tunnel: ["4461: RESET" "Macro: Exit"] -> w179
          frame No Error {
          }
          frame Error {
            w189 = T14 1 items=["no dialog", "OK message", "continue or stop message", "OK message + warnings", "continue/stop + warnings"] ("type of dialog (OK msg:1)")
            # "Unhandled Error -- Display it"
            n92 = call <vilib>:"General Error Handler.vi"("type of dialog (OK msg:1)"=w189, "error in (no error)"=w188) -> ()  [unwired: 9 in, 5 out]
          }
        }
        n93 = call <vilib>:"Add State(s) to Queue__JKI_lib_State_Machine.vi"("State(s) in Front (\"\")"=w179, "State(s) in (\"\")"=w185) -> ("States Out"=w184:string)  [unwired: 13 in]
        "error" <- w177
      }
      frame "Exit" {
        # "Do not put any code in this frame.\n(No errors that occur here will be handled.)"
        n94 = call <vilib>:"Add State(s) to Queue__JKI_lib_State_Machine.vi"("State(s) in (\"\")"=w194) -> ("States Out"=w193:string)  [unwired: 14 in]
      }
      frame "---------- Data ----------" {
        # "Do not put any code in this frame.\n(It is a separator no-op. You can make a copy of this frame to create a new Data frame)"
        n95 = call <vilib>:"Add State(s) to Queue__JKI_lib_State_Machine.vi"("State(s) in (\"\")"=w198) -> ("States Out"=w197:string)  [unwired: 14 in]
      }
      frame "Data: Initialize" {
        w199 = string[] []  # Tasks
        w200 = cluster{"Fs":dbl, "#s":dbl} {"Fs"=204800.0, "#s"=204800.0}  # sampling info
        w201 = waveform(dbl)[] []  # Ouput Signals
        w203 = waveform(dbl)[] []  # Input Signals
        w202 = waveform(dbl)[] []  # REF
        w204 = refnum<k21>[] []  # AO task
        w205 = refnum<k21>[] []  # AI task
        w206 = T15 {"Current VI Reference"=refnum, "Close Panel on Exit?"=FALSE}  # Core
        w208 = FALSE  # Error
        w207 = ""  # Your string data
        # "do not delete - used by framework"
        # "Expand Bundle to add new data elements to shift register data."
        # "Add new data here."
        # "Data names and types of shift register data are defined by this bundle."
        # "Initialize the shift-register data, here.\n(data names are defined by what you wire into the bundle function)"
        n96 = Bundle("Core"=w206, "Error"=w208, "Your string data"=w207, "AI task"=w205, "AO task"=w204, "Input Signals"=w203, "Ouput Signals"=w201, "REF"=w202, "sampling info"=w200, "Tasks"=w199) -> (w210:T13)  [unwired: 1 in]
        n97 = call <vilib>:"Add State(s) to Queue__JKI_lib_State_Machine.vi"("State(s) in (\"\")"=w212) -> ("States Out"=w211:string)  [unwired: 14 in]
      }
      frame "Data: Cleanup" {
        # "Cleanup any data and references, here.\n(this is called automatically, by the Macro: Exit)"
        n98 = Unbundle By Name(w213) -> ("Core.Current VI Reference"=w216:refnum<vi>)
        n99 = Close Reference(reference=w216, error in (no error)=w215) -> (error out=w214:errorcluster)
        n100 = call <vilib>:"Add State(s) to Queue__JKI_lib_State_Machine.vi"("State(s) in (\"\")"=w218) -> ("States Out"=w217:string)  [unwired: 14 in]
      }
      frame "---------- UI ----------" {
        # "Do not put any code in this frame.\n(It is a separator no-op. You can make a copy of this frame to create a new UI frame)"
        n101 = call <vilib>:"Add State(s) to Queue__JKI_lib_State_Machine.vi"("State(s) in (\"\")"=w222) -> ("States Out"=w221:string)  [unwired: 14 in]
      }
      frame "UI: Initialize" {
        w223 = FALSE ("EXIT")
        w227 = waveform(dbl)[][] [] ("History Data")
        # "empty Display charts"
        # "Initialize the User Interface, here.\n(this is called automatically, by the Macro: Init)"
        n102 = local write "error"(errorcluster {"status"=FALSE, "code"=0, "source"=""} ("error out")) -> ()
        n103 = local write "EXIT"(w223) -> ()
        n104 = property on="Display X (or R)" class="WaveformChart (strict)"("History Data"=w227) -> ()  [unwired: 2 in, 2 out]
        n105 = property on="Display Y (or Theta)" class="WaveformChart (strict)"("History Data"=w227) -> ()  [unwired: 2 in, 2 out]
        n106 = local write "RESET"(w223) -> ()
        n107 = local write "Bug"(w223) -> ()
        n108 = call <vilib>:"Add State(s) to Queue__JKI_lib_State_Machine.vi"("State(s) in (\"\")"=w229) -> ("States Out"=w228:string)  [unwired: 14 in]
      }
      frame "UI: Cursor Set" {
        # "Argument"
        # "Set and Unset Cursor Busy.\n(Usage: \"UI: Cursor Set >> Busy|Idle\")"
        n109 = case shown="\"Busy\"" w231 {
          tunnel: w233 -> [w237 w239]
          tunnel: [w236 w238] -> w232
          frame "Idle", Default {
            n110 = call <vilib>:"Unset Busy.vi"("error in (no error)"=w237) -> ("error out"=w236:errorcluster)  [unwired: 10 in]
          }
          frame "Busy" {
            n111 = call <vilib>:"Set Busy.vi"("error in (no error)"=w239) -> ("error out"=w238:errorcluster)  [unwired: 9 in, 1 out]
          }
        }
        n112 = call <vilib>:"Add State(s) to Queue__JKI_lib_State_Machine.vi"("State(s) in (\"\")"=w235) -> ("States Out"=w234:string)  [unwired: 14 in]
      }
      frame "UI: Front Panel State" {
        # "Argument"
        # "Set Front Panel Open or Closed\n(Usage: \"UI: Front Panel State >> Open|Close\")"
        n113 = Unbundle By Name(w241) -> ("Core.Current VI Reference"=w243:refnum<vi>)
        n114 = case shown="\"Open\", Default" w242 {
          tunnel: w244 -> [w250 w263]
          tunnel: [w252 w264] -> w240
          tunnel: w243 -> [w251 w261]
          frame "Open", Default {
            n115 = property class="VI"(reference=w251, error in=w250) -> (reference out=w248:refnum<vi>, error out=w249:errorcluster, "Front Panel.Open"=w247:bool)
            n116 = case shown="True" w247 {
              tunnel: [w255 w258] -> w252
              tunnel: w249 -> [w254 w258]
              tunnel: w248 -> [w253 _]
              frame False {
                n117 = invoke class="VI" method="FP.Open"(reference=w253, error in=w254, "Activate"=TRUE, "State"=T11."Standard") -> (error out=w255:errorcluster)  [unwired: 1 in, 4 out]
              }
              frame True {
              }
            }
          }
          frame "Close" {
            n118 = property class="VI"(reference=w261, error in=w263) -> (reference out=w260:refnum<vi>, error out=w262:errorcluster, "Front Panel.Open"=w259:bool)
            n119 = case shown="True" w259 {
              tunnel: [w265 w268] -> w264
              tunnel: w262 -> [w265 w267]
              tunnel: w260 -> [_ w266]
              frame False {
              }
              frame True {
                n120 = invoke class="VI" method="FP.Close"(reference=w266, error in=w267) -> (error out=w268:errorcluster)  [unwired: 1 in, 2 out]
              }
            }
          }
        }
        n121 = call <vilib>:"Add State(s) to Queue__JKI_lib_State_Machine.vi"("State(s) in (\"\")"=w246) -> ("States Out"=w245:string)  [unwired: 14 in]
      }
      frame "---------- Macro ----------" {
        # "Do not put any code in this frame.\n(It is a separator no-op. You can make a copy of this frame to create a new Macro frame)"
        n122 = call <vilib>:"Add State(s) to Queue__JKI_lib_State_Machine.vi"("State(s) in (\"\")"=w272) -> ("States Out"=w271:string)  [unwired: 14 in]
      }
      frame "Macro: Initialize" {
        w274 = "Data: Initialize\nInitialize Core Data\nUI: Initialize\nUI: Front Panel State >> Open\n#4461: Setup\n#4461: Create Tasks"  # Data: Initialize Initialize Core Data UI: Initialize UI: Front Panel State >> Open #4461: Setup #4461: Create Tasks
        # "Initialization Macro\n(This is called once, when the VI starts)"
        n123 = call <vilib>:"Add State(s) to Queue__JKI_lib_State_Machine.vi"("State(s) in Front (\"\")"=w274, "State(s) in (\"\")"=w277) -> ("States Out"=w276:string)  [unwired: 13 in]
      }
      frame "Macro: Exit" {
        w279 = FALSE ("EXIT")
        # "Exit Macro\n(This is called once, when the VI exits)"
        n124 = Unbundle By Name(w278) -> ("Core.Close Panel on Exit?"=w285:bool)
        n125 = local write "EXIT"(w279) -> ()
        n126 = local write "RESET"(w279) -> ()
        n127 = Select(t="UI: Front Panel State >> Close", s=w285, f="") -> (s? t:f=w282:string)
        n128 = call <vilib>:"Add State(s) to Queue__JKI_lib_State_Machine.vi"("State(s) in (\"\")"=w282, "State(s) at Back (\"\")"="Data: Cleanup\nExit") -> ("States Out"=w280:string)  [unwired: 13 in]
        n129 = call <vilib>:"Add State(s) to Queue__JKI_lib_State_Machine.vi"("State(s) in Front (\"\")"=w280, "State(s) in (\"\")"=w288) -> ("States Out"=w287:string)  [unwired: 13 in]
      }
      frame "---------- 4461----------" {
        n130 = call <vilib>:"Add State(s) to Queue__JKI_lib_State_Machine.vi"("State(s) in (\"\")"=w292) -> ("States Out"=w291:string)  [unwired: 14 in]
      }
      frame "4461: INI" {
        n131 = case shown="True" "save config" {
          tunnel: "Instrument" -> [w310 w314]
          tunnel: w296 -> [w308 w313]
          tunnel: [w307 w312] -> w295
          tunnel: "load config" -> [_ w311]
          frame True {
            n132 = local read "AI Configuration"() -> (w304:T9)
            n133 = local read "AO Configuration"() -> (w305:T8)
            n134 = local read "DAQ Type"() -> (w306:enum16{"None", "USB 4431", "PXI 446x"})
            n135 = local read "Amplifiers"() -> (w303:enum16{"None", "Krohn Hite", "Femto"})
            n136 = call "config.vi"("Function"=enum16{"write", "read"}."write", "Error In"=w308, "Instrument"=w310, "Amplifiers"=w303, "DAQ Type"=w306, "AO Configuration"=w305, "AI Configuration"=w304) -> ("Error Out"=w307:errorcluster)  [unwired: 4 out]
            n137 = local write "save config"(FALSE ("save config")) -> ()
          }
          frame False {
            n138 = case shown="True" w311 {
              tunnel: w314 -> [_ w320]
              tunnel: w313 -> [w315 w318]
              tunnel: [w315 w317] -> w312
              frame False {
              }
              frame True {
                n139 = local write "load config"(FALSE ("load config")) -> ()
                n140 = call "config.vi"("Function"=enum16{"write", "read"}."read", "Error In"=w318, "Instrument"=w320) -> ("Amplifiers"=w323:enum16{"None", "Krohn Hite", "Femto"}, "DAQ Type"=w324:enum16{"None", "USB 4431", "PXI 446x"}, "AO Configuration 2"=w321:T8, "AI Configuration 2"=w322:T9, "Error Out"=w317:errorcluster)  [unwired: 4 in]
                n141 = local write "AI Configuration"(w322) -> ()
                n142 = local write "AO Configuration"(w321) -> ()
                n143 = local write "DAQ Type"(w324) -> ()
                n144 = local write "Amplifiers"(w323) -> ()
              }
            }
          }
        }
        n145 = call <vilib>:"Add State(s) to Queue__JKI_lib_State_Machine.vi"("State(s) in (\"\")"=w299, "State(s) at Back (\"\")"="4461: RESET" ("State(s) at Back (\"\")")) -> ("States Out"=w300:string)  [unwired: 13 in]
      }
      frame "4461: SETUP" {
        n146 = local read "Channels: AO"() -> (w327:T6)
        n147 = Unbundle By Name(w339) -> ("sampling info"=w340:cluster{"Fs":dbl, "#s":dbl})
        n148 = case shown="\"None\"" "DAQ Type" {
          frame "USB 4431", Default {
          }
          frame "PXI 446x" {
          }
          frame "None" {
            n149 = local write "Amplifiers"(enum16{"None", "Krohn Hite", "Femto"}."None" ("Amplifiers")) -> ()
          }
        }
        n150 = case shown="\"None\"" "DAQ Type" {
          tunnel: [u32 0 u32 0 u32 16448250] -> w335
          tunnel: [u32 6618880 u32 6618880 u32 16711680] -> w334
          frame "USB 4431" {
          }
          frame "PXI 446x" {
          }
          frame "None" {
          }
        }
        n151 = Unbundle By Name(w327) -> ("AO f (Hz)"=w325:dbl[])
        n152 = Index Array(array=w325) -> (element=w329:dbl)  [unwired: 1 in]
        n153 = property on="DAQ mode string" class="Str"("Text.BG Color"=w334, "Text.FG Color"=w335) -> ()  [unwired: 2 in, 2 out]
        n154 = property on="DAQ Type" class="Enum (strict)"() -> ("RingText.Text"=→"DAQ mode string":string)  [unwired: 2 in, 2 out]
        n155 = Bundle(cluster=cluster{"Fs":i32, "#s":i32} {"Fs"=204000, "#s"=34} ("sampling info"), "Fs"="Fs", "#s"="#s") -> (w330:cluster{"Fs":i32, "#s":i32})
        "sampling info" <- w330
        n156 = case shown="True" "auto size" {
          tunnel: w340 -> [_ w365]
          tunnel: [w351 w366] -> w338
          tunnel: w329 -> [_ w352]
          tunnel: "DAQ Type" -> [_ w359]
          tunnel: w330 -> [w351 _]
          frame False {
          }
          frame True {
            n157 = case shown="\"USB 4431\", Default" w359 {
              tunnel: [102400.0 ("upper limit") 204800.0 ("upper limit") 204800.0 ("upper limit")] -> w353
              frame "USB 4431", Default {
              }
              frame "PXI 446x" {
              }
              frame "None" {
              }
            }
            n158 = Multiply(x="frequency multiplier", y=w352) -> (x*y=w364:dbl)
            n159 = In Range and Coerce(upper limit=w353, x=w364, lower limit=1000.0) -> (coerced(x)=w362:dbl)  [unwired: 1 out]
            n160 = call "Fs and Ns for integer periods.vi"("f_integer"=w352, "Fs"=w362) -> ("#s_integer"=w355:dbl, "Fs_integer"=w357:dbl)  [unwired: 8 in]
            n161 = In Range and Coerce(upper limit=w353, x=w355, lower limit=128.0) -> (coerced(x)=w354:dbl)  [unwired: 1 out]
            n162 = In Range and Coerce(upper limit=w353, x=w357, lower limit=1000.0) -> (coerced(x)=w358:dbl)  [unwired: 1 out]
            n163 = local write "#s"(w354) -> ()
            n164 = Bundle By Name(cluster=w365, "Fs"=w358, "#s"=w354) -> (w366:cluster{"Fs":dbl, "#s":dbl})
            n165 = local write "Fs"(w358) -> ()
          }
        }
        n166 = Bundle By Name(cluster=w339, "sampling info"=w338) -> (w337:T13)
        n167 = call <vilib>:"Add State(s) to Queue__JKI_lib_State_Machine.vi"("State(s) in (\"\")"=w343) -> ("States Out"=w342:string)  [unwired: 14 in]
      }
      frame "4461: CREATE TASKS" {
        w377 = 10178 items=["Finite Samples"=10178, "Continuous Samples"=10123] ("sample mode")
        w376 = 10123 items=["Finite Samples"=10178, "Continuous Samples"=10123] ("sample mode")
        n168 = local read "AO Configuration"() -> (w381:T8)
        n169 = local read "Channels: Lockin"() -> (w374:T7)
        n170 = local read "AI Configuration"() -> (w383:T9)
        n171 = local read "AI Buffer Size (S)"() -> (w388:i32)
        n172 = Unbundle By Name(w378) -> ("sampling info"=w379:cluster{"Fs":dbl, "#s":dbl})
        n173 = local read "Channels: AO"() -> (w389:T6)
        n174 = local read "DAQ Type"() -> (w373:enum16{"None", "USB 4431", "PXI 446x"})
        n175 = local read "IV Curve Mode"() -> (w370:bool)
        n176 = Equal?(x=w373, y=enum16{"None", "USB 4431", "PXI 446x"}."None" ("DAQ Type")) -> (x = y?=w371:bool)
        n177 = Select(t=w377, s=w370, f=w376) -> (s? t:f=w375:i32)
        n178 = case shown="False" w371 {
          tunnel: w383 -> [w403 _]
          tunnel: w381 -> [w402 _]
          tunnel: [w401 w422] -> w387
          tunnel: w379 -> [w400 w419]
          tunnel: [w399 w422] -> w386
          tunnel: w388 -> [w398 _]
          tunnel: [w397 dbl[] [] ("phase log")] -> w382
          tunnel: w389 -> [w396 w420]
          tunnel: w384 -> [w395 w425]
          tunnel: [w394 w424] -> w380
          tunnel: w375 -> [w393 _]
          tunnel: w374 -> [w392 w421]
          tunnel: w370 -> [_ w418]
          frame False {
            n179 = disable-structure shown="Default" {
              disable-tunnel: w403 -> [w415 _]
              disable-tunnel: w402 -> [w414 _]
              disable-tunnel: [w413 _] -> w401
              disable-tunnel: w400 -> [w410 _]
              disable-tunnel: [w412 _] -> w399
              disable-tunnel: w398 -> [w408 _]
              disable-tunnel: [w409 _] -> w397
              disable-tunnel: w396 -> [w411 _]
              disable-tunnel: w395 -> [w407 _]
              disable-tunnel: [w406 _] -> w394
              disable-tunnel: w393 -> [w405 _]
              disable-tunnel: w392 -> [w404 _]
              frame condition #0 (active) {
                n180 = call "4431 USB - Create IO Channels.vi"("sample mode"=w405, "Channels: Lockin"=w404, "error in"=w407, "AI Buffer Size (S)"=w408, "sampling info"=w410, "AO"=w411, "AO Configuration"=w414, "AI Configuration"=w415) -> ("AO Task"=w412:refnum<k21>[], "AI task"=w413:refnum<k21>[], "error out"=w406:errorcluster, "phase log"=w409:dbl[])
              }
              frame condition #1 {
              }
            }
          }
          frame True {
            w422 = refnum<k21>[] [] ("AI task")
            # "simulate mode"
            n181 = Not(x=w418) -> (.not. x?=w417:bool)
            n182 = Initialize Array(1.0 ("element"), 8 ("dimension size")) -> (w416:dbl[])
            n183 = call "4461 - Create AO waveforms.vi"("sampling info"=w419, "reset signal"=w417, "AO"=w420) -> ()  [unwired: 5 in, 4 out]
            n184 = call "4461 - Create Reference Waveforms.vi"("sampling info"=w419, "reset signal"=w417, "Lockin"=w421) -> ()  [unwired: 5 in, 4 out]
            n185 = call <userlib>:"FGV - KH Gain.vi"("error in"=w425, "Function"=enum16{"write", "read"}."write", "Array"=w416) -> ("error out"=w424:errorcluster)  [unwired: 3 in, 1 out]
            n186 = local write "Gain"(w416) -> ()
          }
        }
        n187 = local write "phase log"(w382) -> ()
        n188 = Bundle By Name(cluster=w378, "AI task"=w387, "AO task"=w386) -> (w385:T13)
        n189 = call <vilib>:"Add State(s) to Queue__JKI_lib_State_Machine.vi"("State(s) in (\"\")"=w391) -> ("States Out"=w390:string)  [unwired: 14 in]
      }
      frame "4461: READ WRITE" {
        n190 = Unbundle By Name(w459) -> ("sampling info"=w442:cluster{"Fs":dbl, "#s":dbl}, "AI task"=w458:refnum<k21>[])
        n191 = local read "IV Curve Mode"() -> (w429:bool)
        n192 = local read "..........reset signal"() -> (w431:bool)
        n193 = local read "....measure offset"() -> (w457:bool)
        n194 = local read "Channels: AO"() -> (w451:T6)
        n195 = Unbundle By Name(w451) -> ("AO amp (V)"=w448:dbl[])
        n196 = Array Size(array=w448) -> (size(s)=w449:i32)
        n197 = Initialize Array(0.0 ("element"), w449) -> (w446:dbl[])
        n198 = local read "Channels: Lockin"() -> (w455:T7)
        n199 = Bundle By Name(cluster=w451, "AO amp (V)"=w446) -> (w450:T6)
        n200 = Get Date/Time In Seconds() -> (seconds since 1Jan1904=w439:timestamp)
        n201 = Select(t=FALSE, s=w429, f=w431) -> ()  [unwired: 1 out]
        n202 = Format Date/Time String(time format string (%c)="%H:%M:%S%1u   %Y-%m-%d", seconds (now)=w439) -> (date/time string=→"time and date":string)  [unwired: 1 in]
        n203 = Select(t=w450, s=w457, f=w451) -> (s? t:f=w456:T6)
        n204 = Or(x=w429, y=w431) -> (x .or. y?=w430:bool)
        n205 = call "4461 - Create AO waveforms.vi"("error in (no error)"=w469, "sampling info"=w442, "reset signal"=w430, "AO"=w456) -> ("error out"=w454:errorcluster, "phase out"=w452:dbl[], "AO Array"=w453:waveform(dbl)[])  [unwired: 4 in, 1 out]
        n206 = call "4461 - Create Reference Waveforms.vi"("error in (no error)"=w469, "sampling info"=w442, "reset signal"=w430, "Lockin"=w455) -> ("error out"=w461:errorcluster, "AO Array"=w445:waveform(dbl)[])  [unwired: 4 in, 2 out]
        n207 = local read "DAQ Type"() -> (w441:enum16{"None", "USB 4431", "PXI 446x"})
        n208 = call-poly <userlib>:"Empty Array__ogtk.vi"("Array"=w458) -> ("Empty Array?"=w434:bool)  [unwired: 8 in]
        n209 = local write "phase log"(w452) -> ()
        n210 = Equal?(x=w441, y=enum16{"None", "USB 4431", "PXI 446x"}."None" ("DAQ Type")) -> (x = y?=w440:bool)
        n211 = Or(x=w434, y=w440) -> (x .or. y?=w435:bool)
        n212 = case shown="False" w435 {
          tunnel: [w489 w503] -> w443
          tunnel: w453 -> [w483 w501]
          tunnel: w442 -> [w484 w500]
          tunnel: w459 -> [w486 _]
          tunnel: w454 -> [w485 w502]
          tunnel: [w487 w502] -> w468
          tunnel: [w482 w501] -> w444
          tunnel: w429 -> [w480 _]
          frame False {
            n213 = Unbundle By Name(w486) -> ("AI task"=w488:refnum<k21>[], "AO task"=w481:refnum<k21>[])
            n214 = disable-structure shown="Default" {
              disable-tunnel: [w491 _] -> w489
              disable-tunnel: w483 -> [w492 w498]
              disable-tunnel: w484 -> [w493 _]
              disable-tunnel: w488 -> [w495 _]
              disable-tunnel: w485 -> [w497 _]
              disable-tunnel: [w496 _] -> w487
              disable-tunnel: [w492 w498] -> w482
              disable-tunnel: w481 -> [w494 _]
              disable-tunnel: w480 -> [w490 _]
              frame condition #0 (active) {
                n215 = call "4461 - AI AND AI - Read AND Write Uneven -- Array.vi"("Reset"=w490, "AO Array"=w492, "error in (no error)"=w497, "sampling info"=w493, "AO Task"=w494, "AI task"=w495) -> ("error out"=w496:errorcluster, "Input Signals"=w491:waveform(dbl)[])  [unwired: 4 in]
              }
              frame condition #1 {
              }
            }
            n216 = property on="DAQ mode string" class="Str"("Text.BG Color"=u32 6618880) -> ()  [unwired: 2 in, 2 out]
          }
          frame True {
            n217 = call "4461 Sim - Noise.vi"("data"=w501, "sampling info"=w500) -> ("Data"=w503:waveform(dbl)[])  [unwired: 5 in]
            n218 = local write "DAQ Type"(enum16{"None", "USB 4431", "PXI 446x"}."None" ("DAQ Type")) -> ()
          }
        }
        n219 = case shown="True" w434 {
          frame False {
          }
          frame True {
            # "flash colors to alert user"
            n220 = property on="DAQ mode string" class="Str"() -> ("Text.BG Color"=w475:u32)  [unwired: 2 in, 2 out]
            n221 = Equal?(x=w475, y=u32 16711680) -> (x = y?=w474:bool)
            n222 = case shown="False" w474 {
              tunnel: [u32 16711680 u32 16448250] -> w473
              frame False {
              }
              frame True {
              }
            }
            n223 = property on="DAQ mode string" class="Str"("Text.BG Color"=w473) -> ()  [unwired: 2 in, 2 out]
          }
        }
        n224 = Index Array(array=w443) -> (element=w466:waveform(dbl))  [unwired: 1 in]
        n225 = local write "time since trigger"(0.0 ("time since trigger")) -> ()
        n226 = Unbundle By Name(w466) -> ("Y"=w465:dbl[])
        n227 = Bundle By Name(cluster=w459, "Input Signals"=w443, "Ouput Signals"=w444, "REF"=w445) -> (w470:T13)
        n228 = call-poly <userlib>:"Empty Array__ogtk.vi"("Array"=w465) -> ("Empty Array?"=w463:bool)  [unwired: 8 in]
        n229 = Merge Errors(w468, w461) -> (w467:errorcluster)
        n230 = Select(t="4461: RESET" ("State(s) at Back (\"\")"), s=w463, f="" ("State(s) at Back (\"\")")) -> (s? t:f=w432:string)
        n231 = call <vilib>:"Add State(s) to Queue__JKI_lib_State_Machine.vi"("State(s) in Front (\"\")"=w432, "State(s) in (\"\")"=w472) -> ("States Out"=w471:string)  [unwired: 13 in]
      }
      frame "4461: FILTER" {
        w506 = TRUE ("averaging")
        n232 = Unbundle By Name(w508) -> ("Ouput Signals"=w505:waveform(dbl)[], "Input Signals"=w527:waveform(dbl)[], "REF"=w517:waveform(dbl)[])
        n233 = local read "decimating factor"() -> (w510:i32)
        n234 = call "decimate_waveforms.vi"("decimating factor"=w510, "averaging"=w506, "error in (no error)"=w522, "Input Signal"=w505) -> ("error out"=w521:errorcluster, "Decimated Waveforms"=w504:waveform(dbl)[])  [unwired: 6 in]
        n235 = call "decimate_waveforms.vi"("decimating factor"=w510, "averaging"=w506, "error in (no error)"=w522, "Input Signal"=w527) -> ("error out"=w524:errorcluster, "Decimated Waveforms"=w515:waveform(dbl)[])  [unwired: 6 in]
        n236 = call "decimate_waveforms.vi"("decimating factor"=w510, "averaging"=w506, "error in (no error)"=w522, "Input Signal"=w517) -> ("error out"=w523:errorcluster, "Decimated Waveforms"=w509:waveform(dbl)[])  [unwired: 6 in]
        n237 = local read "offsets"() -> (w528:dbl[])
        n238 = Subtract(x=w515, y=w528) -> (x-y=w514:waveform(dbl)[])
        n239 = Merge Errors(w521, w524, w523) -> (w519:errorcluster)
        n240 = case shown="False" "60 Hz prefilter" {
          tunnel: w514 -> [w536 w538]
          tunnel: [w536 w537] -> w513
          frame False {
          }
          frame True {
            n241 = call "Prefilter_60Hz_Notch.vi"("Array"=w538) -> ("Array 2"=w537:waveform(dbl)[])  [unwired: 10 in]
          }
        }
        n242 = local read "............zero offset"() -> (w518:bool)
        n243 = local read "....measure offset"() -> (w520:bool)
        n244 = Index Array(array=w509) -> (element=w526:waveform(dbl))  [unwired: 1 in]
        n245 = case shown="False" "LP prefilter" {
          tunnel: w513 -> [w532 w535]
          tunnel: [w532 w534] -> w512
          tunnel: "LP cutoff (Hz)" -> [_ w533]
          frame False {
          }
          frame True {
            n246 = call "Prefilter_LP.vi"("high cutoff freq [Hz]"=w533, "Array"=w535) -> ("Array 2"=w534:waveform(dbl)[])  [unwired: 9 in]
          }
        }
        n247 = Unbundle By Name(w526) -> ("dt"=w525:dbl)
        n248 = local write "dt"(w525) -> ()
        n249 = case shown="False" w520 {
          tunnel: w508 -> [w542 w547]
          frame False {
            n250 = Unbundle By Name(w542) -> ("Input Signals"=w541:waveform(dbl)[])
            n251 = for {
              tunnel: w541 -> [w544] mode=indexing
              tunnel: [w543] -> w540 mode=indexing
              n252 = call-poly <vilib>:"Mean.vi"("X"=w544) -> ("mean"=w543:dbl)  [unwired: 1 out]
            }
            n253 = local write "mean"(w540) -> ()
          }
          frame True {
            n254 = Unbundle By Name(w547) -> ("Input Signals"=w546:waveform(dbl)[])
            n255 = for {
              tunnel: w546 -> [w549] mode=indexing
              tunnel: [w548] -> w545 mode=indexing
              n256 = call-poly <vilib>:"Mean.vi"("X"=w549) -> ("mean"=w548:dbl)  [unwired: 1 out]
            }
            n257 = local write "offsets"(w545) -> ()
            n258 = local write "mean"(w545) -> ()
          }
        }
        n259 = case shown="False" w518 {
          frame False {
          }
          frame True {
            n260 = local write "offsets"(dbl[] [0.0, 0.0, 0.0, 0.0, 0.0, 0.0, 0.0, 0.0] ("offsets")) -> ()
          }
        }
        n261 = Bundle By Name(cluster=w508, "Ouput Signals"=w504, "Input Signals"=w512, "REF"=w509) -> (w529:T13)
        n262 = call <vilib>:"Add State(s) to Queue__JKI_lib_State_Machine.vi"("State(s) in (\"\")"=w531) -> ("States Out"=w530:string)  [unwired: 14 in]
      }
      frame "4461: PHASE" {
        n263 = local read "Results\n(X, Y, R, Theta, mean)"() -> (w561:dbl[][])
        n264 = local read "autophase?\n(experimental)"() -> (w560:bool)
        n265 = local read "phase log"() -> (w562:dbl[])
        n266 = local read "Channels: Lockin"() -> (w558:T7)
        n267 = local read "Channels: AO"() -> (w557:T6)
        n268 = call "lockin - Set all f same.vi"("all  frequencies same?"="............all  f same", "Lockin"=w558, "AO"=w557) -> ("Lockin 2"=w555:T7, "AO 2"=w554:T6)  [unwired: 7 in]
        n269 = call "lockin - Set REF phase equals zero.vi"("reset REF phi to zero"="...............reset REF", "Channels: Lockin"=w555, "Channels: AO"=w554) -> ("Channels: Lockin 2"=w550:T7, "Channels: AO 2"=w556:T6)  [unwired: 7 in]
        n270 = case shown="True" w560 {
          tunnel: w562 -> [_ w571]
          tunnel: w561 -> [_ w570]
          tunnel: w550 -> [w566 w568]
          tunnel: [w566 w567] -> w551
          frame False {
          }
          frame True {
            # "do this for EACH lockin...\n- replace PID array with PID SV\n-  advance \"results\" by 8?\n- this should go BEFORE REF\nwaveform is generated"
            n271 = Index Array(array=w570, index (col)=3 ("index (row)")) -> (element=w573:dbl[])  [unwired: 1 in]
            n272 = call "Simple PID Array.vi"("D"="D", "I"="I", "P"="P", "process variable"=w573) -> ("output value"=w577:dbl[])  [unwired: 7 in]
            n273 = Subtract(x=w571, y=w577) -> (x-y=w569:dbl[])
            n274 = Bundle By Name(cluster=w568, "REF phi (deg)"=w569) -> (w567:T7)
          }
        }
        n275 = local write "Channels: AO"(w556) -> ()
        n276 = local write "Channels: Lockin"(w551) -> ()
        n277 = call <vilib>:"Add State(s) to Queue__JKI_lib_State_Machine.vi"("State(s) in (\"\")"=w565) -> ("States Out"=w564:string)  [unwired: 14 in]
      }
      frame "4461: LOCKIN" {
        (unwired) 0
        # "Display stuff and lockin calculations"
        n278 = Unbundle By Name(w626) -> ("Ouput Signals"=w582:waveform(dbl)[], "Input Signals"=w600:waveform(dbl)[], "REF"=w581:waveform(dbl)[], "sampling info"=w590:cluster{"Fs":dbl, "#s":dbl})
        n279 = local read "TC (s)"() -> (w624:dbl)
        n280 = local read "mean"() -> (w618:dbl[])
        n281 = local read "order"() -> (w623:i32)
        n282 = local read "Gain"() -> (w588:dbl[])
        n283 = local read "Gain"() -> (w587:dbl[])
        n284 = Select(t="applied signals (V)" ("Y Scale.Name Label.Text"), s="Output signals?", f="REF signal (arb)" ("Y Scale.Name Label.Text")) -> (s? t:f=w589:string)
        n285 = Select(t=w582, s="Output signals?", f=w581) -> (s? t:f=w596:waveform(dbl)[])
        n286 = Divide(x=w600, y=w587) -> (x/y=w585:waveform(dbl)[])
        n287 = property on="Reference Graph" class="WFGraph (strict)"("YScale.NameLbl.Text"=w589) -> ()  [unwired: 2 in, 2 out]
        n288 = Divide(x=w618, y=w588) -> (x/y=w617:dbl[])
        n289 = call "Display n or dt.vi"("Display n?"="Display n?", "Input Waveforms"=w600) -> ("Output Waveforms"=w604:waveform(dbl)[])  [unwired: 9 in]
        n290 = call "Display n or dt.vi"("Display n?"="Display n?", "Input Waveforms"=w596) -> ("Output Waveforms"=w602:waveform(dbl)[])  [unwired: 9 in]
        n291 = call "decimate_waveforms.vi"("decimating factor"="decimate graph", "averaging"=FALSE, "Input Signal"=w602) -> ("Decimated Waveforms"=→"Reference Graph":waveform(dbl)[])  [unwired: 7 in, 1 out]
        n292 = call "decimate_waveforms.vi"("decimating factor"="decimate graph", "averaging"=FALSE, "Input Signal"=w604) -> ("Decimated Waveforms"=→"Signals Graph":waveform(dbl)[])  [unwired: 7 in, 1 out]
        n293 = call "4461 - Lockin Engine.vi"("order"=w623, "TC (s)"=w624, "sampling info"=w590, "Reference In"=w581, "Signal in"=w585) -> ("filter fC (Hz)"=w594:dbl, "Results (X,Y,R,Theta)"=w620:dbl[][])  [unwired: 5 in]
        n294 = Transpose 2D Array(2D array=w620) -> (transposed array=w613:dbl[][])
        n295 = Build Array (concatenate)(w613, w617) -> (w619:dbl[][])
        n296 = Index Array(array=w585) -> (element=w597:waveform(dbl))  [unwired: 1 in]
        n297 = call "FGV - Signals - Output.vi"("Function"=enum16{"write", "read"}."write", "input signal"=w582) -> ()  [unwired: 4 in, 2 out]
        n298 = call "FGV - Signals - Input.vi"("Function"=enum16{"write", "read"}."write", "input signal"=w585) -> ()  [unwired: 4 in, 2 out]
        n299 = local read "Channel"() -> (w595:dbl)
        n300 = local write "filter fC (Hz)"(w594) -> ()
        n301 = local read "Display"() -> (w622:enum16{"X and Y", "R and Theta"})
        n302 = Transpose 2D Array(2D array=w619) -> (transposed array=w601:dbl[][])
        "Results\n(X, Y, R, Theta, mean)" <- w601
        n303 = Unbundle By Name(w597) -> ("t0"=w584:timestamp)
        n304 = local read "Tab Control 2"() -> (w616:T1)
        n305 = call "format display.vi"("Channel"=w595, "Display"=w622, "Results (X,Y,R,Theta)"=w620, "t0"=w584) -> ("X/R"=→"X or R":dbl, "Array 2"=→"XY Graph":cluster{dbl[], dbl[]}[], "Y/Theta Array"=→"Display Y (or Theta)":waveform(dbl)[], "X/R Array"=→"Display X (or R)":waveform(dbl)[], "Y/R"=→"Y or Theta":dbl)  [unwired: 3 in]
        n306 = call "FGV - Lockin Results.vi"("Function"=enum16{"write", "read"}."write", "Input Signals"=w601) -> ()  [unwired: 4 in, 2 out]
        n307 = Equal?(x=w616, y=T12."PS" ("Tab Control 2")) -> (x = y?=w583:bool)
        n308 = Select(t="4461: FFT" ("State(s) at Back (\"\")"), s=w583, f="" ("State(s) at Back (\"\")")) -> (s? t:f=w579:string)
        n309 = call <vilib>:"Add State(s) to Queue__JKI_lib_State_Machine.vi"("State(s) in (\"\")"=w628, "State(s) at Back (\"\")"=w579) -> ("States Out"=w625:string)  [unwired: 13 in]
      }
      frame "4461: FFT" {
        n310 = Unbundle By Name(w649) -> ("Input Signals"=w631:waveform(dbl)[])
        n311 = local read "Gain"() -> (w647:dbl[])
        n312 = Divide(x=w631, y=w647) -> (x/y=w638:waveform(dbl)[])
        n313 = call-poly <vilib>:"FFT Power Spectrum and PSD.vi"("window parameter"="window parameter", "export mode"="export mode", "averaging parameters"="averaging parameters", "restart averaging (F)"="restart averaging (F)", "dB On (F)"=TRUE, "window"="window", "time signals"=w638) -> ("averages completed"=→"averages\ncompleted":dbl, "averaging done"=→"averaging done":bool, "Power Spectrum / PSD"=w629:cluster{"f0":dbl, "df":dbl, "magnitude":dbl[]}[])  [unwired: 1 in, 1 out]
        "PS dB" <- w629
        n314 = for {
          tunnel: w629 -> [w669] mode=indexing
          tunnel: [w664] -> w630 mode=indexing
          n315 = Unbundle By Name(w669) -> ("df"=w671:dbl, "magnitude"=w670:dbl[])  [unwired: 1 out]
          n316 = Bundle By Name("dt"=w671, "Y"=w670) -> (w668:waveform(dbl))  [unwired: 1 in]
          n317 = call-poly <vilib>:"Waveform to XY Pairs.vi"("waveform in"=w668) -> ("XY pairs"=w667:cluster{"x":timestamp, "y":dbl}[])  [unwired: 8 in, 2 out]
          n318 = for {
            tunnel: w667 -> [w675] mode=indexing
            tunnel: [w673] -> w665 mode=indexing
            tunnel: [w672] -> w666 mode=indexing
            n319 = Unbundle(w675) -> ("x"=w674:timestamp, "y"=w673:dbl)
            n320 = To Double Precision Float(number=w674) -> (double precision float=w672:dbl)
          }
          n321 = Bundle(w666, w665) -> (w664:cluster{dbl[], dbl[]})  [unwired: 1 in]
        }
        n322 = property on="PS dB" class="WFGraph (strict)"("Active Cursor"=u32 1) -> ("Cursor.Cursor X"=w643:dbl)  [unwired: 2 in, 2 out]
        n323 = property on="PS dB" class="WFGraph (strict)"("Active Cursor"=u32 0) -> ("Cursor.Cursor X"=w644:dbl)  [unwired: 2 in, 2 out]
        n324 = Build Array(w644, w643) -> (w642:dbl[])
        n325 = for {
          tunnel: w630 -> [w663] mode=indexing
          tunnel: w642 -> [w662]
          tunnel: [w654] -> w641 mode=indexing
          n326 = Array Max & Min(array=w662) -> (max value=w661:dbl, min value=w659:dbl)  [unwired: 2 out]
          n327 = Unbundle(w663) -> (w660:dbl[], w658:dbl[])
          n328 = Threshold 1D Array(2:w661, 3:w660) -> (0:w657:dbl)  [unwired: 1 in]
          n329 = Threshold 1D Array(2:w659, 3:w660) -> (0:w656:dbl)  [unwired: 1 in]
          n330 = Subtract(x=w657, y=w656) -> (x-y=w655:dbl)
          n331 = Array Subset(array=w658, index=w656, length=w655) -> (w653:dbl[])
          n332 = Add Array Elements(numeric array=w653) -> (sum=w654:dbl)
        }
        n333 = Build Array(w641) -> (→"PS Chart":dbl[][])
        n334 = call <vilib>:"Add State(s) to Queue__JKI_lib_State_Machine.vi"("State(s) in (\"\")"=w652) -> ("States Out"=w650:string)  [unwired: 14 in]
      }
      frame "4461: SAVE" {
        w678 = "FFT" ("filename")
        w677 = "signal" ("filename")
        # "Wait for Trigger signal from other VI"
        n335 = local read "PS dB"() -> (w694:cluster{"f0":dbl, "df":dbl, "magnitude":dbl[]}[])
        n336 = Get Date/Time In Seconds() -> (seconds since 1Jan1904=w685:timestamp)
        n337 = local read "Path"() -> (w676:path)
        n338 = for {
          tunnel: w694 -> [w714] mode=indexing
          tunnel: [w709] -> w689 mode=indexing
          n339 = Unbundle By Name(w714) -> ("df"=w716:dbl, "magnitude"=w715:dbl[])  [unwired: 1 out]
          n340 = Bundle By Name("dt"=w716, "Y"=w715) -> (w713:waveform(dbl))  [unwired: 1 in]
          n341 = call-poly <vilib>:"Waveform to XY Pairs.vi"("waveform in"=w713) -> ("XY pairs"=w712:cluster{"x":timestamp, "y":dbl}[])  [unwired: 8 in, 2 out]
          n342 = for {
            tunnel: w712 -> [w720] mode=indexing
            tunnel: [w718] -> w710 mode=indexing
            tunnel: [w717] -> w711 mode=indexing
            n343 = Unbundle(w720) -> ("x"=w719:timestamp, "y"=w718:dbl)
            n344 = To Double Precision Float(number=w719) -> (double precision float=w717:dbl)
          }
          n345 = Bundle(w711, w710) -> (w709:cluster{dbl[], dbl[]})  [unwired: 1 in]
        }
        n346 = call "FGV - Signals - Input.vi"("error in"=w686, "Function"=enum16{"write", "read"}."read") -> ("error out"=w687:errorcluster, "input signal"=w693:waveform(dbl)[])  [unwired: 4 in]
        n347 = for {
          tunnel: [w701] -> w692 mode=indexing
          tunnel: w693 -> [w700] mode=indexing
          n348 = call-poly <vilib>:"Waveform to XY Pairs.vi"("waveform in"=w700) -> ("XY pairs"=w704:cluster{"x":timestamp, "y":dbl}[])  [unwired: 8 in, 2 out]
          n349 = for {
            tunnel: w704 -> [w708] mode=indexing
            tunnel: [w706] -> w702 mode=indexing
            tunnel: [w705] -> w703 mode=indexing
            n350 = Unbundle(w708) -> ("x"=w707:timestamp, "y"=w706:dbl)
            n351 = To Double Precision Float(number=w707) -> (double precision float=w705:dbl)
          }
          n352 = Bundle(w703, w702) -> (w701:cluster{dbl[], dbl[]})  [unwired: 1 in]
        }
        n353 = Format Date/Time String(time format string (%c)="%Y-%m-%d", seconds (now)=w685) -> (date/time string=w683:string)  [unwired: 1 in]
        n354 = Build Path(base path=w676, name or relative path=w683) -> (appended path=w681:path)
        n355 = Build Path(base path=w681, name or relative path=w677) -> (appended path=w680:path)
        n356 = call <userlib>:"LV to ITX XY AutoPlot.vi"("filename"=w677, "path"=w680, "Notes"="Notes", "XY Array"=w692, "wavenames (.Vx, etc)"=string[] ["ch0", "ch1", "ch2", "ch3", "ch4", "ch5", "ch6", "ch7"]) -> ()  [unwired: 10 in, 1 out]
        n357 = Build Path(base path=w681, name or relative path=w678) -> (appended path=w679:path)
        n358 = local write "Save Data"(FALSE ("SAVE DATA")) -> ()
        n359 = call <userlib>:"LV to ITX XY AutoPlot.vi"("filename"=w678, "path"=w679, "Notes"="Notes", "XY Array"=w689, "wavenames (.Vx, etc)"=string[] ["FFT0", "FFT1", "FFT2", "FFT3", "FFT4", "FFT5", "FFT6", "FFT7"], "X,Y Log"=i32[] [1, 1]) -> ()  [unwired: 9 in, 1 out]
        n360 = call <vilib>:"Add State(s) to Queue__JKI_lib_State_Machine.vi"("State(s) in (\"\")"=w699) -> ("States Out"=w698:string)  [unwired: 14 in]
      }
      frame "4461: STOP TASKS" {
        w723 = refnum<k21>[] [] ("AI task")
        w721 = FALSE ("Trigger")
        n361 = Unbundle By Name(w725) -> ("AI task"=w734:refnum<k21>[], "AO task"=w738:refnum<k21>[])
        n362 = local read "DAQ Type"() -> (w731:enum16{"None", "USB 4431", "PXI 446x"})
        n363 = call-poly <userlib>:"Empty Array__ogtk.vi"("Array"=w734) -> ("Empty Array?"=w733:bool)  [unwired: 8 in]
        n364 = Equal?(x=w731, y=enum16{"None", "USB 4431", "PXI 446x"}."None" ("DAQ Type")) -> (x = y?=w730:bool)
        n365 = Or(x=w730, y=w733) -> (x .or. y?=w732:bool)
        n366 = case shown="False" w732 {
          tunnel: w738 -> [w742 _]
          tunnel: w736 -> [w741 w770]
          tunnel: [w740 w770] -> w727
          tunnel: w734 -> [w739 _]
          frame False {
            n367 = disable-structure shown="Default" {
              disable-tunnel: w742 -> [w744 _]
              disable-tunnel: w741 -> [w745 _]
              disable-tunnel: [w746 _] -> w740
              disable-tunnel: w739 -> [w743 _]
              frame condition #0 (active) {
                n368 = for {
                  tunnel: w744 -> [w769] mode=indexing
                  tunnel: [w767] -> w751 mode=indexing
                  tunnel: w745 -> [w766]
                  tunnel: [w765] -> w748
                  n369 = call <vilib>:"DAQmx Stop Task.vi"("task/channels in"=w769, "error in"=w766) -> ("task out"=w767:refnum<k21>, "error out"=w765:errorcluster)  [unwired: 12 in]
                  n370 = Wait (ms)(milliseconds to wait=u32 50) -> ()  [unwired: 1 out]
                }
                n371 = for {
                  tunnel: w743 -> [w764] mode=indexing
                  tunnel: [w762] -> w747 mode=indexing
                  tunnel: w748 -> [w761]
                  tunnel: [w760] -> w750
                  n372 = call <vilib>:"DAQmx Stop Task.vi"("task/channels in"=w764, "error in"=w761) -> ("task out"=w762:refnum<k21>, "error out"=w760:errorcluster)  [unwired: 12 in]
                  n373 = Wait (ms)(milliseconds to wait=u32 50) -> ()  [unwired: 1 out]
                }
                n374 = for {
                  tunnel: w751 -> [w759] mode=indexing
                  tunnel: w750 -> [w757]
                  tunnel: [w756] -> w749
                  n375 = call <vilib>:"DAQmx Clear Task.vi"("task in"=w759, "error in"=w757) -> ("error out"=w756:errorcluster)  [unwired: 13 in]
                  n376 = Wait (ms)(milliseconds to wait=u32 50) -> ()  [unwired: 1 out]
                }
                n377 = for {
                  tunnel: w747 -> [w755] mode=indexing
                  tunnel: w749 -> [w753]
                  tunnel: [w752] -> w746
                  n378 = call <vilib>:"DAQmx Clear Task.vi"("task in"=w755, "error in"=w753) -> ("error out"=w752:errorcluster)  [unwired: 13 in]
                  n379 = Wait (ms)(milliseconds to wait=u32 50) -> ()  [unwired: 1 out]
                }
              }
              frame condition #1 {
              }
            }
          }
          frame True {
          }
        }
        n380 = local write "RESET"(FALSE ("EXIT")) -> ()
        n381 = local write "Trigger"(w721) -> ()
        n382 = Bundle By Name(cluster=w725, "AI task"=w723, "AO task"=w723) -> (w724:T13)
        n383 = call <vilib>:"Add State(s) to Queue__JKI_lib_State_Machine.vi"("State(s) in (\"\")"=w737) -> ("States Out"=w722:string)  [unwired: 14 in]
        n384 = call "FGV - Trigger.vi"("error in"=w727, "Function"=enum16{"write", "read"}."write", "Trigger"=w721) -> ("error out"=w726:errorcluster)  [unwired: 3 in, 1 out]
      }
      frame "4461: RESET" {
        n385 = call <vilib>:"Add State(s) to Queue__JKI_lib_State_Machine.vi"("State(s) in Front (\"\")"="4461: STOP TASKS", "State(s) in (\"\")"=w775) -> ("States Out"=w771:string)  [unwired: 13 in]
      }
    }
    n386 = call "StateHistory.vi"("Current State in"=w3) -> ("Current State out"=→"Current State":string, "delimited string"=→"State History":string)  [unwired: 9 in]
  }
